vi "PvgeneratorOP600.vi"(8 "errin":errorcluster, 10 "network":path, 11 "path in":path) -> (0 "sortie d'erreur":errorcluster caption="errout", 1 "network out":path, 2 "tout bon":bool, 3 "Chaîne":string)   [LabVIEW 2020]
uses:
  VG/IS30%.vi
  VG/PN.vi
  SubVI/OP600ZP_VGConf.vi
panel:
  out "Tab1":string[][](array[string])
  out "nombre de remplacements":i32
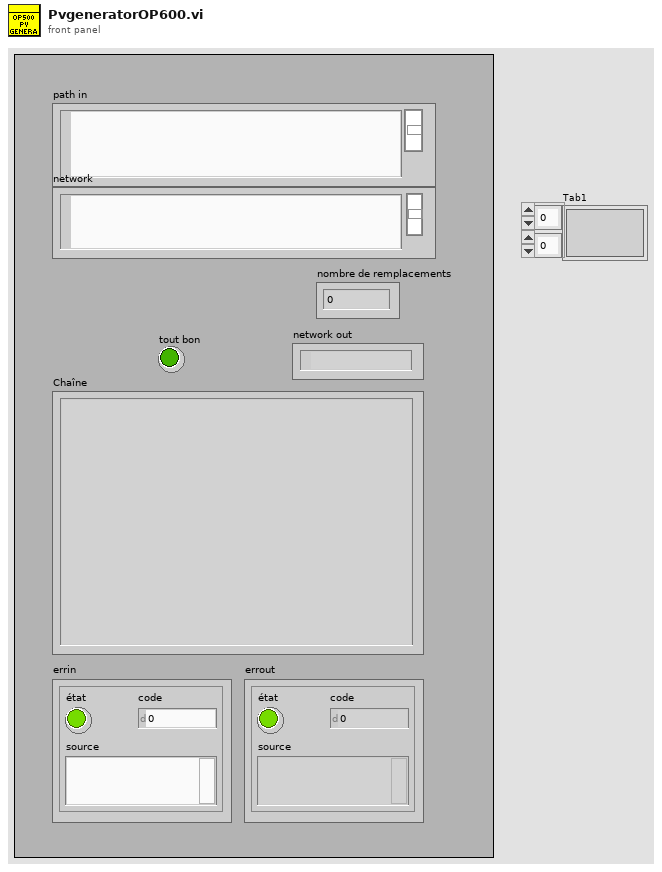
[diagram p1: front panel]
types:
  T1 = enum16{"open", "replace", "create", "open or create", "replace or create", "replace or create with confirmation"}
  T2 = cluster{string, string, string, string, string, string, string, string, string, string}
  T3 = cluster{string, string, string, string, string, string, string, string}
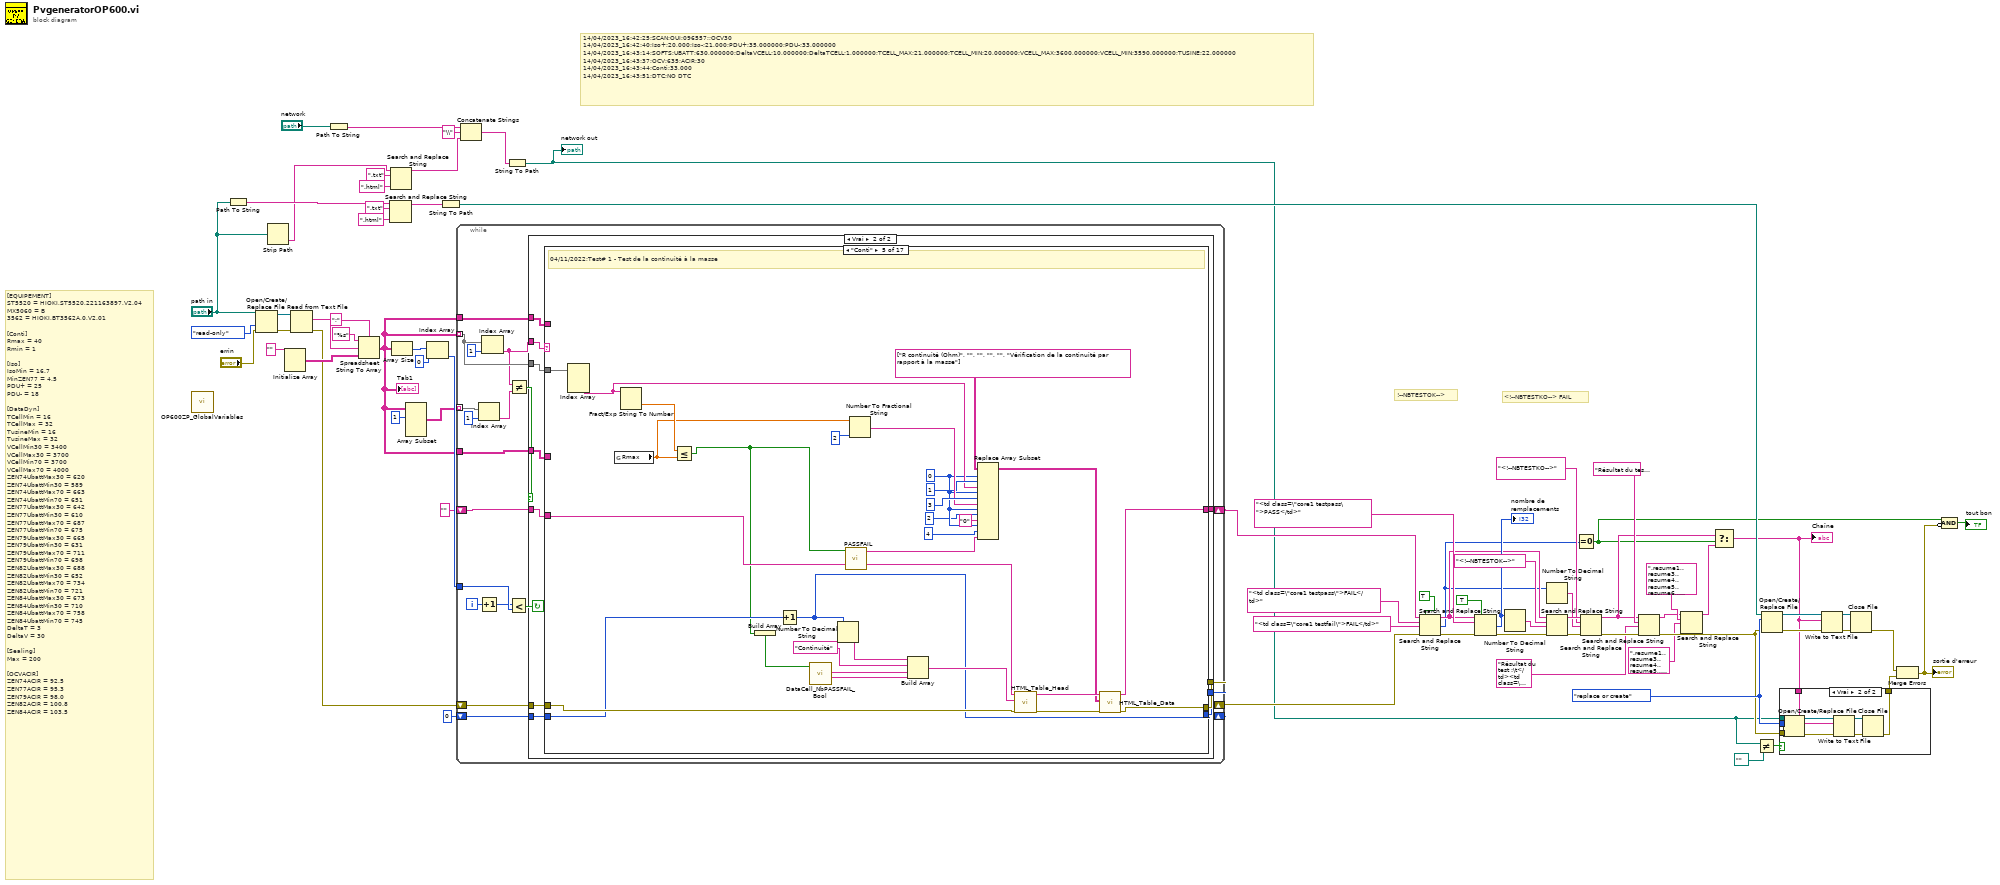
[diagram p0: block diagram]
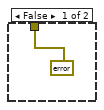
[diagram p2: hidden frame]
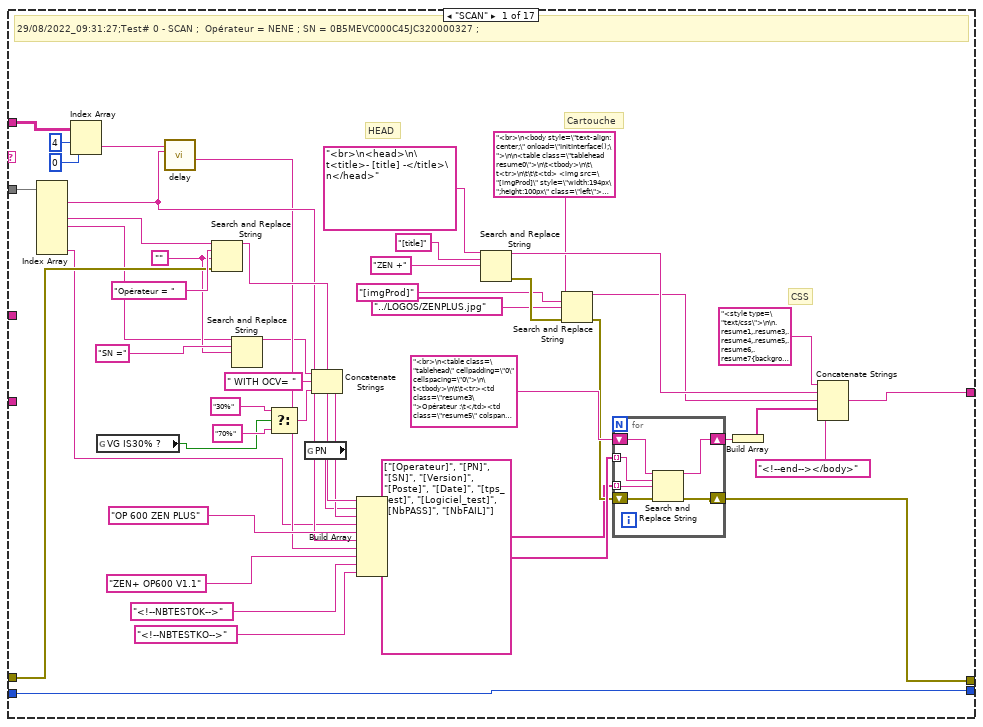
[diagram p4: hidden frame]
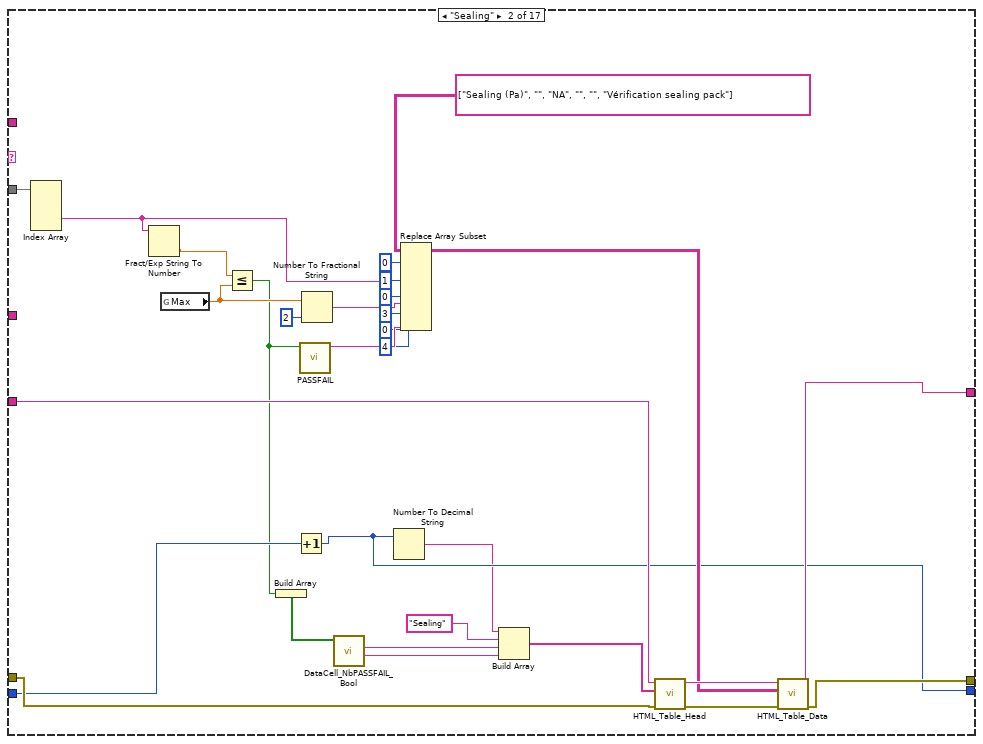
[diagram p5: hidden frame]
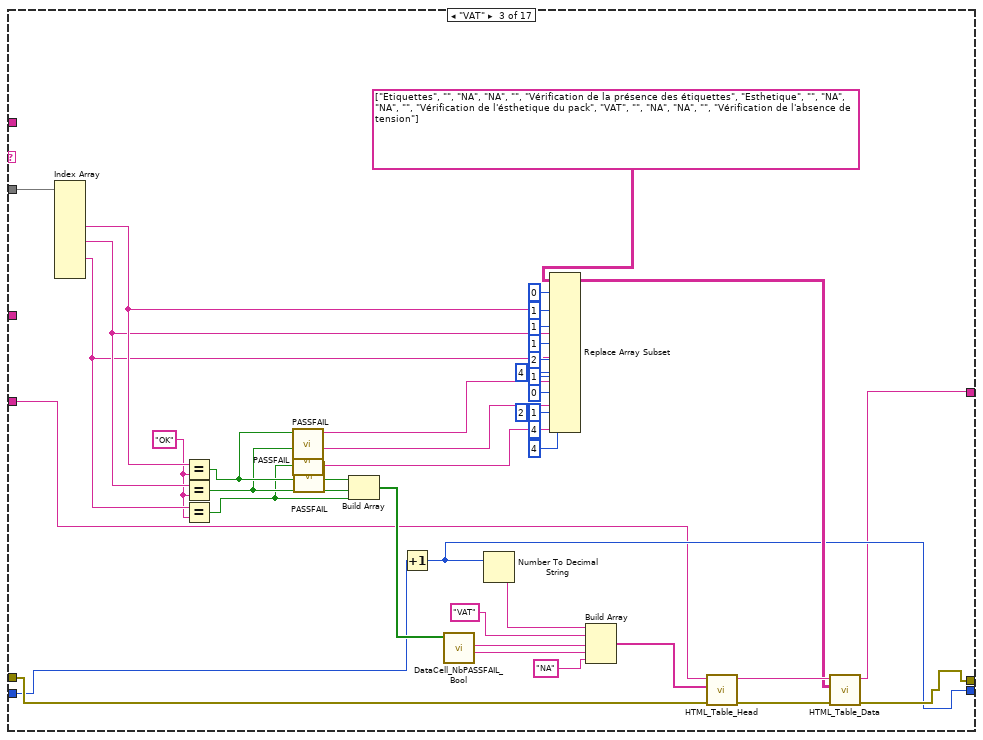
[diagram p6: hidden frame]
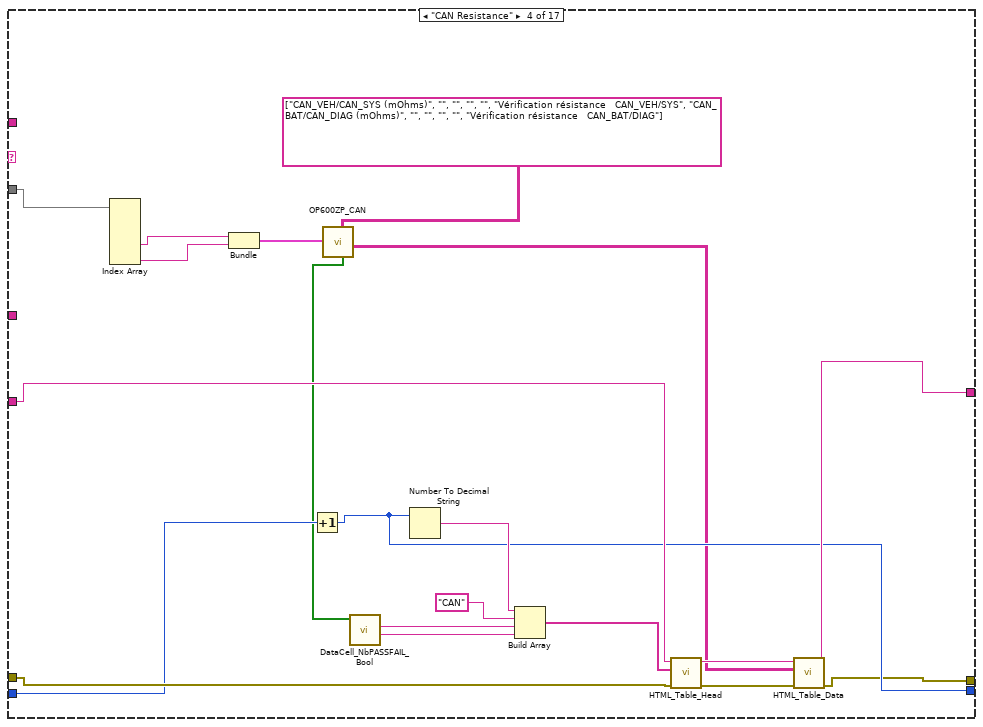
[diagram p7: hidden frame]
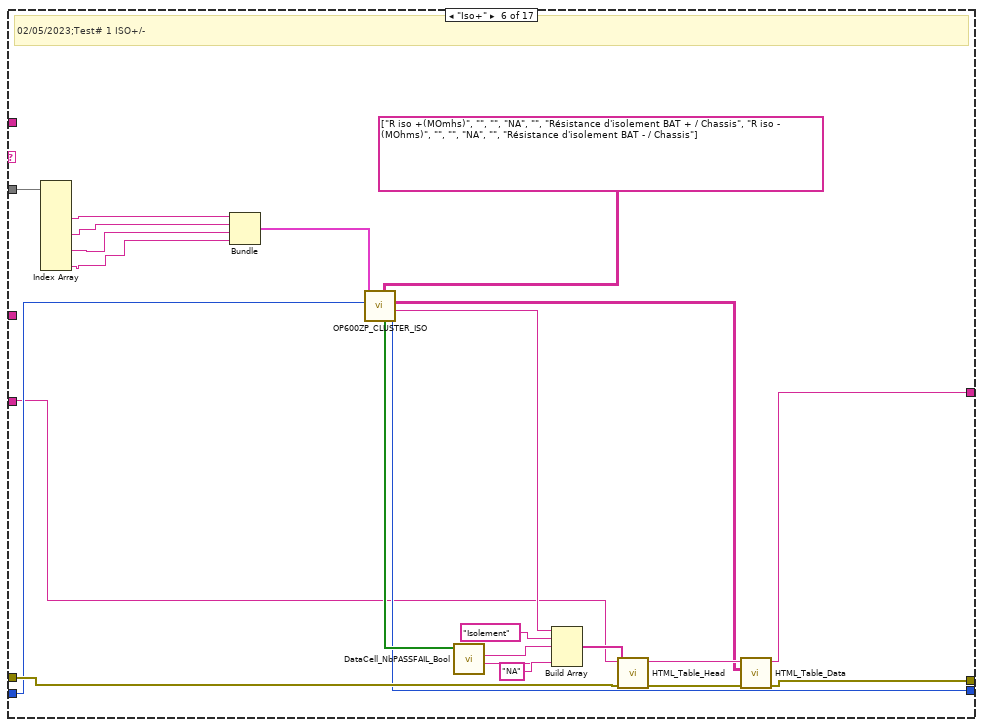
[diagram p8: hidden frame]
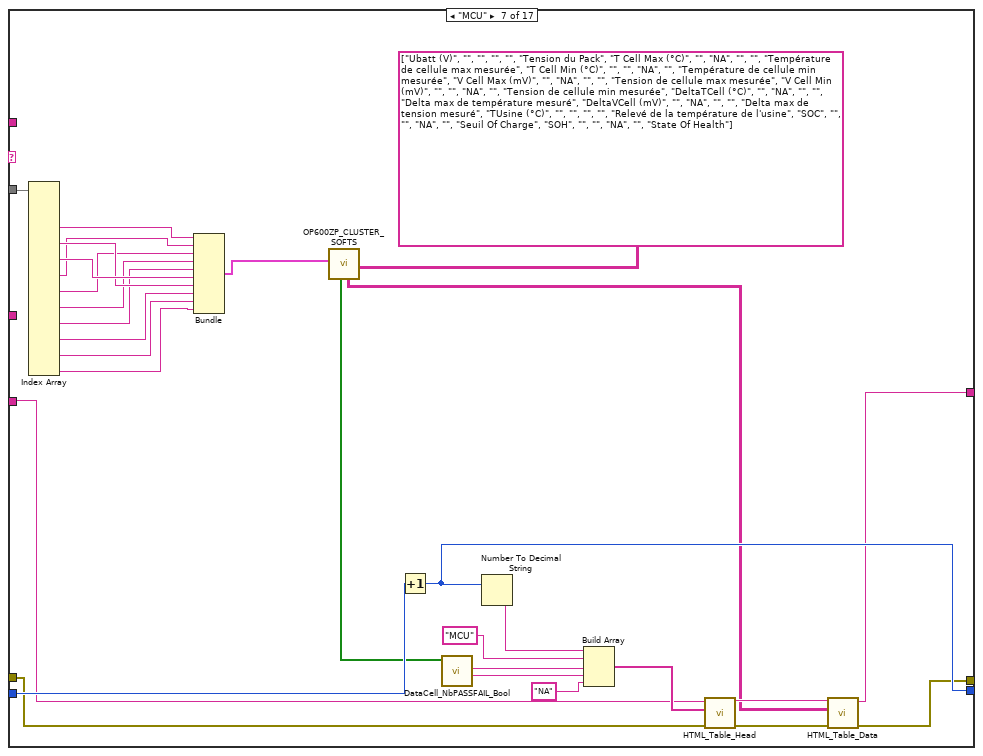
[diagram p9: hidden frame]
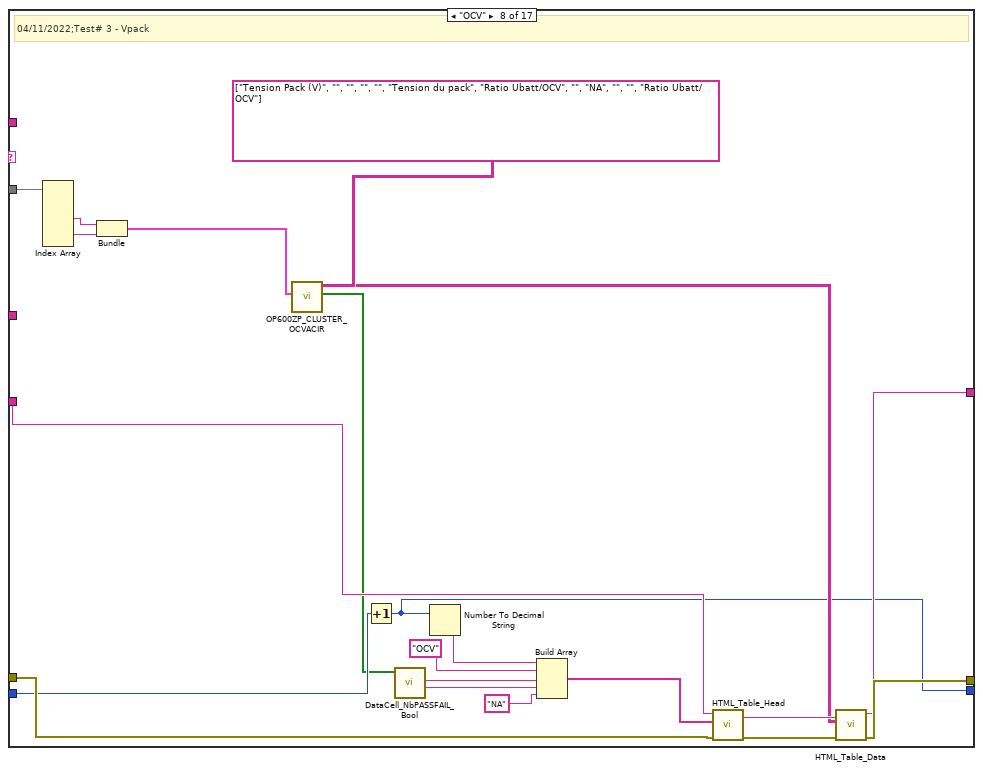
[diagram p10: hidden frame]
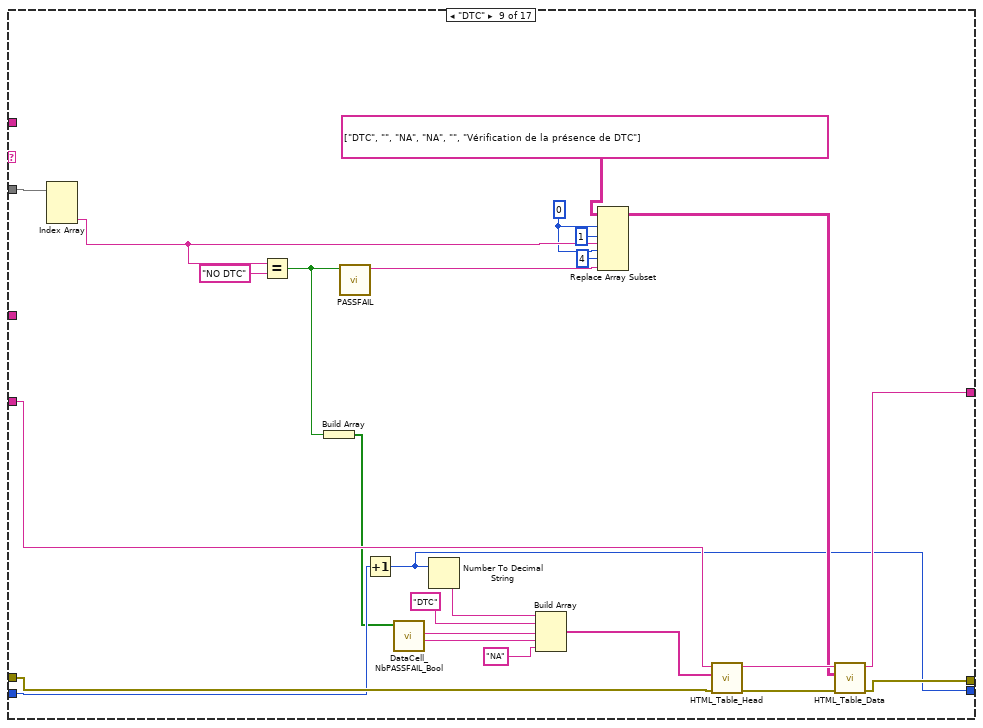
[diagram p11: hidden frame]
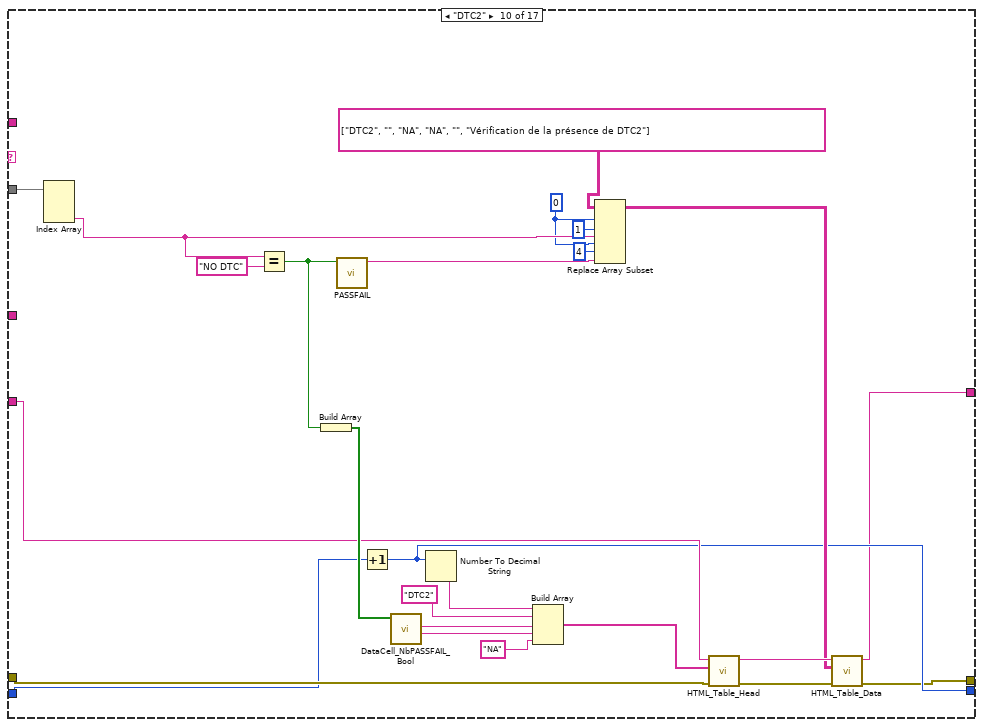
[diagram p12: hidden frame]
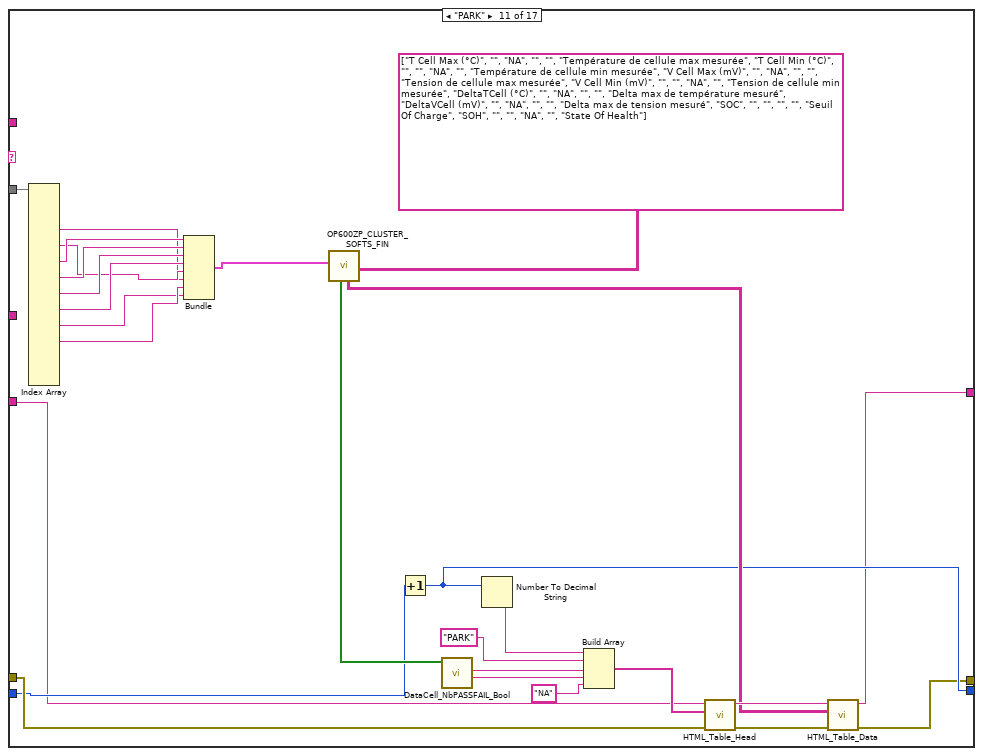
[diagram p13: hidden frame]
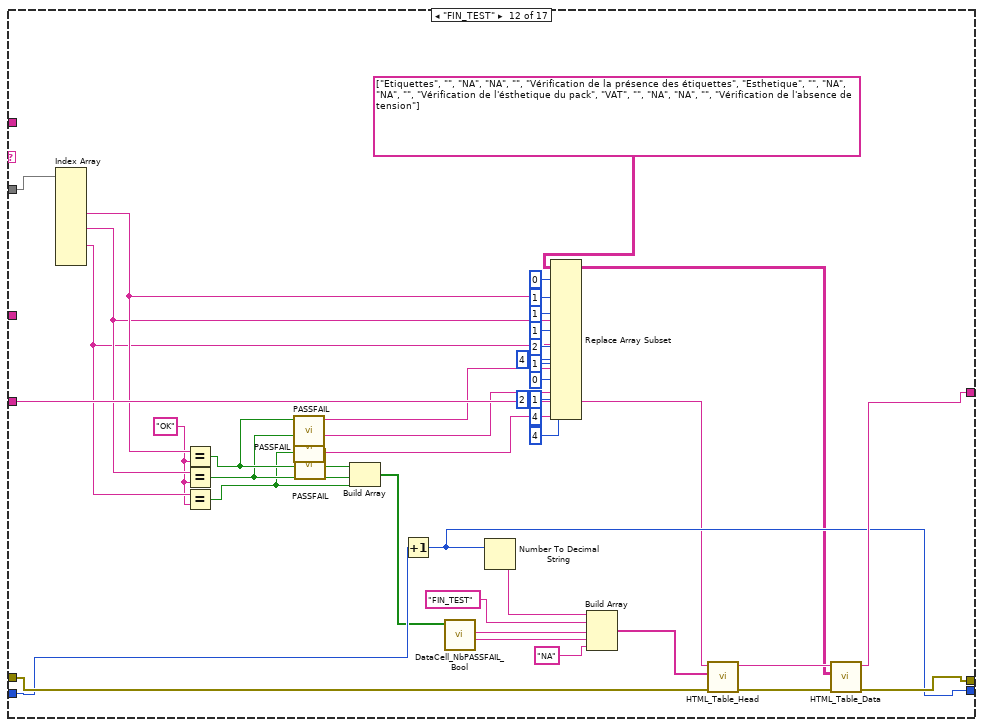
[diagram p14: hidden frame]
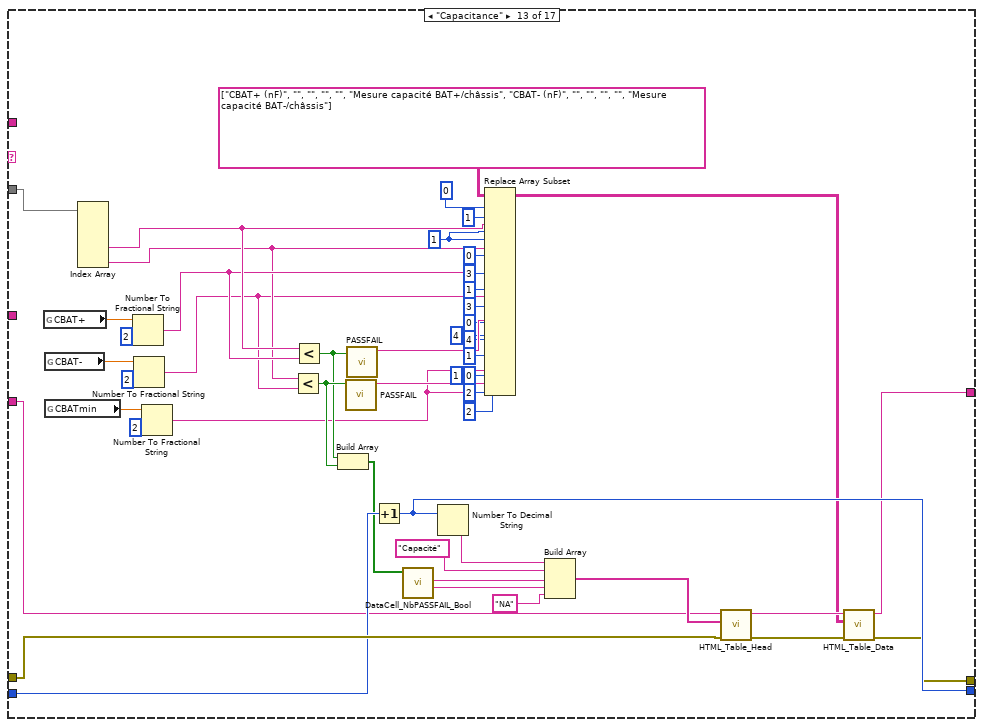
[diagram p15: hidden frame]
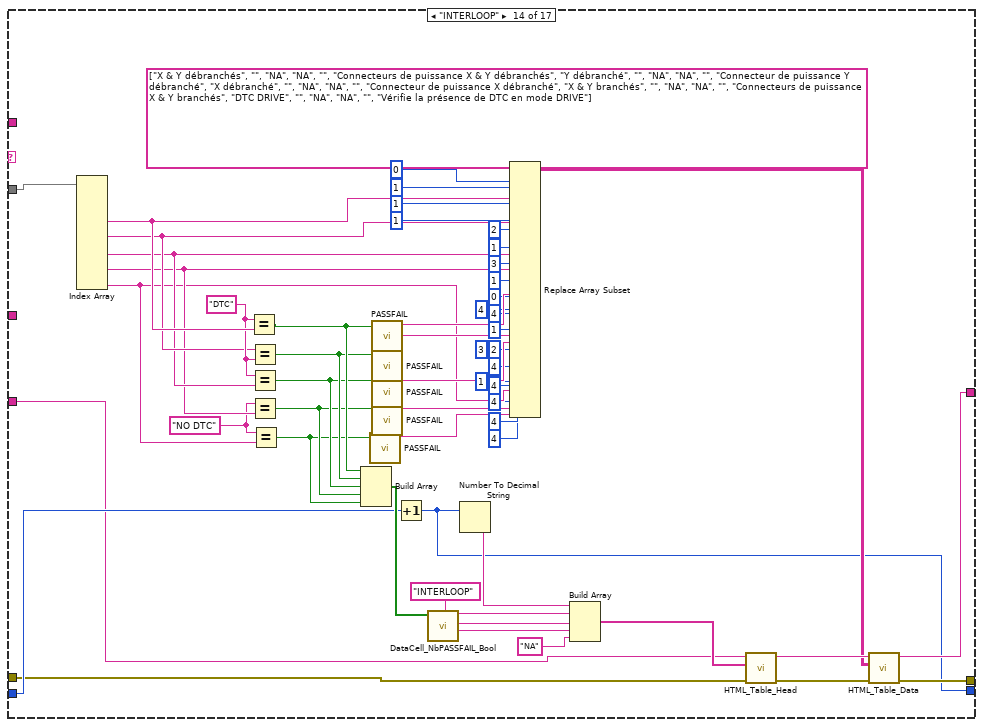
[diagram p16: hidden frame]
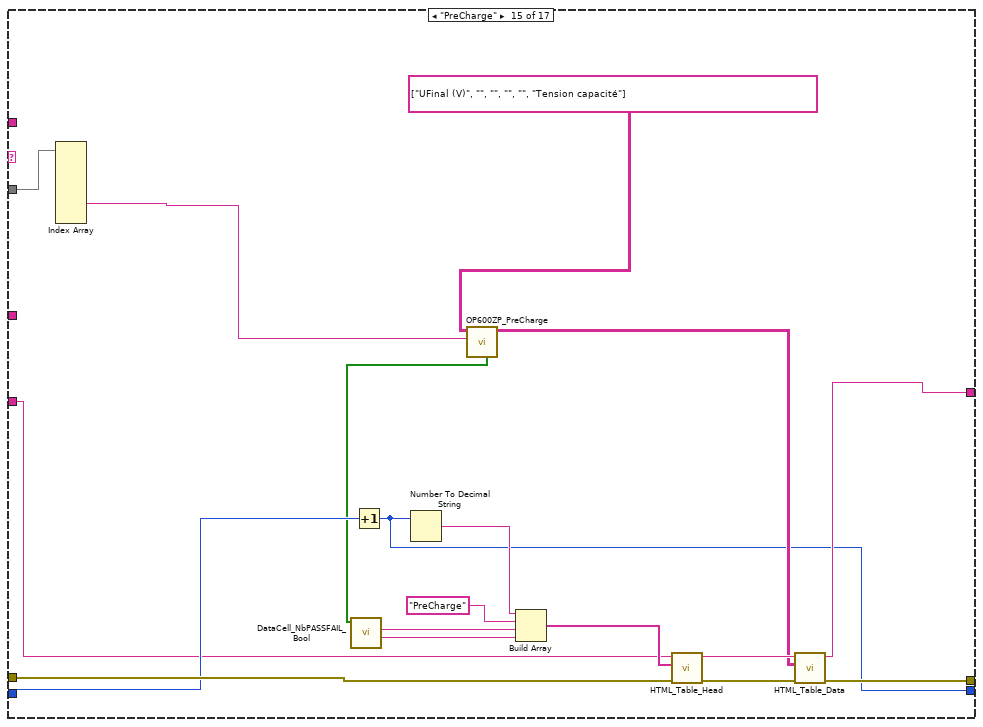
[diagram p17: hidden frame]
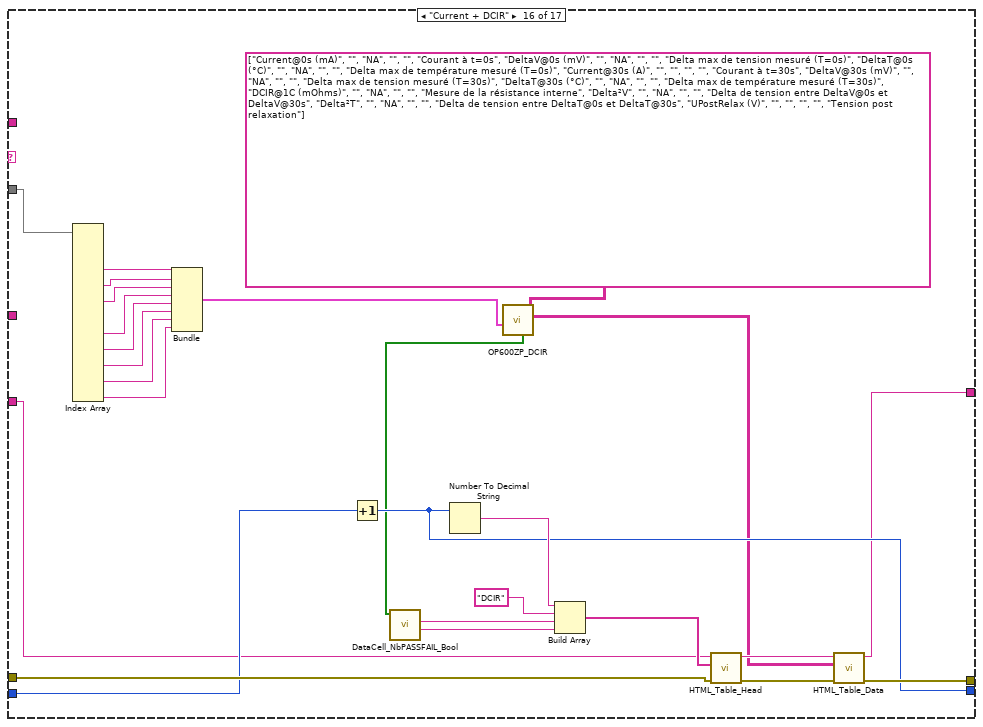
[diagram p18: hidden frame]
diagram:
  w32 = T1."replace or create" ("opération (0 : open)")
  # "14/04/2023_16:42:25;SCAN;OUI;096557;;OCV30\n14/04/2023_16:42:40;Iso+;20,000;Iso-;21,000;PDU+;35,000000;PDU-;33,000000\n14/04/2023_16:43:14;SOFTS;UBATT;630,000000;DeltaVCELL;10,000000;DeltaTCELL;1,000000;TCELL_MAX;21,000000;TCELL_MIN;20,000000;VCELL_MAX;3600,000000;VCELL_MIN;3590,000000;TUSINE;22,000000\n14/04/2023_16:43:37;OCV;635;ACIR;30\n14/04/2023_16:43:44;Conti;33,000\n14/04/2023_16:43:51;DTC;NO DTC"
  # "[EQUIPEMENT]\nST5520 = HIOKI,ST5520,221163897,V2.04\t\nMX5060 = B\n3562 = HIOKI,BT3562A,0,V2.01\n\n[Conti]\nRmax = 40\nRmin = 1\n\n[Iso]\nIsoMin = 16.7\nMinZEN77 = 4.5\nPDU+ = 25\nPDU- = 18\n\n[DataDyn]\nTCellMin = 16\nTCellMax = 32\nTusineMin = 16\nTusineMax = 32\nVCellMin30 = 3400\nVCellMax30 = 3700\nVCellMin70 = 3700\nVCellMax70 = 4000\nZEN74UbattMax30 = 620\nZEN74UbattMin30 = 589\nZEN74UbattMax70 = 663\nZEN74UbattMin70 = 651\nZEN77UbattMax30 = 642\nZEN77UbattMin30 = 610\nZEN77UbattMax70 = 687\nZEN77UbattMin70 = 675\nZEN79UbattMax30 = 665\nZEN79UbattMin30 = 631\nZEN79UbattMax70 = 711\nZEN79UbattMin70 = 698\nZEN82UbattMax30 = 688\nZEN82UbattMin30 = 652\nZEN82UbattMax70 = 734\nZEN82UbattMin70 = 721\nZEN84UbattMax30 = 673\nZEN84UbattMin30 = 710\nZEN84UbattMax70 = 758\nZEN84UbattMin70 = 745\nDeltaT = 3\nDeltaV = 30\n\n[Sealing]\nMax = 200\n\n[OCVACIR]\nZEN74ACIR = 92.5\nZEN77ACIR = 95.3\nZEN79ACIR = 98.0\nZEN82ACIR = 100.8\nZEN84ACIR = 103.5"
  # "<!--NBTESTKO--> FAIL"
  # "!--NBTESTOK-->"
  n1 = call "OP600ZP_GlobalVariables.vi"() -> ()  [unwired: 12 in]
  n2 = Path To String(path="path in") -> (string=w54:string)
  n3 = Open/Create/Replace File(file path (use dialog)="path in", error in="errin", access (0:read/write)=enum16{"read/write", "read-only", "write-only"}."read-only" ("accès (0 : read/write)")) -> (refnum out=w55:refnum<file>, error out=w72:errorcluster)  [unwired: 3 in, 1 out]
  n4 = Strip Path(path="path in") -> (name=w13:string)  [unwired: 1 out]
  n5 = Initialize Array("") -> (w70:string[][])  [unwired: 2 in]
  n6 = Read from Text File(file (use dialog)=w55, error in=w72) -> (text=w68:string, error out=w60:errorcluster)  [unwired: 2 in, 2 out]
  n7 = Path To String(path="network") -> (string=w12:string)
  n8 = Spreadsheet String To Array(delimiter (Tab)=";" ("séparateur (Tabulation)"), format string="%s" ("chaîne de format"), spreadsheet string=w68, array type (2D Dbl)=w70) -> (array=w3:string[][])
  "Tab1" <- w3
  n9 = Search and Replace String(input string=w54, search string=".txt" ("chaîne recherchée"), replace string=".html" ("chaîne de remplacement (\"\")")) -> (result string=w51:string)  [unwired: 5 in, 3 out]
  n10 = Search and Replace String(input string=w13, search string=".txt" ("chaîne recherchée"), replace string=".html" ("chaîne de remplacement (\"\")")) -> (result string=w10:string)  [unwired: 5 in, 3 out]
  n11 = Array Size(array=w3) -> (size(s)=w66:i32[])
  n12 = Array Subset(array=w3, index (row)=1 ("indice")) -> (w1:string[][])  [unwired: 3 in]
  n13 = Index Array(array=w66, index=0 ("indice")) -> (element=w64:i32)
  n14 = String To Path(string=w51) -> (path=w50:path)
  n15 = while {
    tunnel: w64 -> [w91]
    tunnel: w3 -> [w88] mode=indexing
    shift-right: [w87] -> w47
    shift-left: w60 -> [w86]
    shift-right: [w80] -> w49
    shift-left: "" -> [w85]
    shift-right: [w83] -> _
    shift-left: 0 -> [w84]
    tunnel: w3 -> [w82]
    tunnel: w3 -> [w79]
    tunnel: w1 -> [w77] mode=indexing
    i -> [w92]
    stop <- w90 continue-if-true
    n16 = Index Array(array=w77, index=1 ("indice")) -> (element=w76:string)
    n17 = Increment(x=w92) -> (x+1=w81:i32)
    n18 = Index Array(array=w88, index=1 ("indice")) -> (element=w75:string)
    n19 = Less?(x=w81, y=w91) -> (x < y?=w90:bool)
    n20 = Not Equal?(x=w75, y=w76) -> (x != y?=w74:bool)
    n21 = case shown="Vrai" w74 {
      tunnel: w88 -> [_ w105]
      tunnel: [w94 w97] -> w87
      tunnel: w86 -> [w94 w104]
      tunnel: w85 -> [w95 w103]
      tunnel: w84 -> [w93 w102]
      tunnel: [w93 w96] -> w83
      tunnel: w82 -> [_ w101]
      tunnel: [w95 w98] -> w80
      tunnel: w75 -> [_ w100]
      tunnel: w79 -> [_ w99]
      frame False {
      }
      frame True {
        n22 = case shown="\"Conti\"" w100 {
          tunnel: w104 -> [w150 w182 w192 w241 w271 w294 w318 w343 w368 w383 w416 w458 w504 w527 w580 w607 w618]
          tunnel: w105 -> [w152 w188 w189 w235 w272 w295 w330 w344 w361 w381 w417 w468 w516 w571 w589 w615 _]
          tunnel: [w129 w181 w195 w236 w270 w293 w316 w342 w367 w378 w412 w457 w499 w529 w575 w606 w618] -> w97
          tunnel: w103 -> [_ w175 w193 w238 w269 w285 w315 w341 w362 w380 w414 w453 w501 w526 w578 w593 w616]
          tunnel: w102 -> [w128 w177 w191 w240 w268 w292 w322 w340 w366 w382 w415 w454 w503 w528 w579 w605 w617]
          tunnel: [w128 w174 w194 w237 w267 w286 w321 w331 w352 w379 w413 w455 w502 w525 w574 w604 w617] -> w96
          tunnel: w101 -> [_ _ _ _ _ _ _ _ _ _ _ _ _ _ _ _ _]
          tunnel: w99 -> [w121 _ _ _ _ _ _ _ _ _ _ _ _ _ _ _ _]
          tunnel: [w127 w176 w190 w239 w266 w291 w320 w339 w363 w377 w411 w456 w498 w530 w576 w602 w616] -> w98
          frame "SCAN" {
            w123 = ""
            # "Cartouche"
            # "HEAD"
            # "CSS"
            # "29/08/2022_09:31:27;Test# 0 - SCAN ;  Opérateur = NENE ; SN = 0B5MEVC000C45JC320000327 ;"
            n23 = Index Array(array=w152) -> (element #1=w117:string, element #3=w126:string, element #4=w122:string, element #7=w106:string)  [unwired: 7 in, 3 out]
            n24 = Index Array(array=w121, index (row)=4, index (col)=0 ("disabled index (col)")) -> (element=w118:string)
            n25 = global read "IS30%.vi" "VG IS30% ?"() -> (w108:bool)
            n26 = call "delay.vi"("String"=w117, "String 2"=w118) -> ("Delay calculé"=w116:string)  [unwired: 9 in]
            n27 = Search and Replace String(input string=w126, search string="Opérateur = " ("chaîne recherchée"), replace string=w123, error in=w150) -> (result string=w125:string)  [unwired: 4 in, 3 out]
            n28 = Search and Replace String(input string=w122, search string="SN =" ("chaîne recherchée"), replace string=w123) -> (result string=w114:string)  [unwired: 5 in, 3 out]
            n29 = Select(t="30%" ("y"), s=w108, f="70%" ("y")) -> (s? t:f=w111:string)
            n30 = global read "PN.vi" "PN"() -> (w107:string)
            n31 = Concatenate Strings(w114, " WITH OCV= " ("chaîne"), w111) -> (w113:string)
            n32 = Build Array(w125, w107, w113, w106, "OP 600 ZEN PLUS" ("chaîne"), w117, w116, "ZEN+ OP600 V1.1" ("chaîne"), "<!--NBTESTOK-->" ("chaîne"), "<!--NBTESTKO-->" ("chaîne")) -> (w130:string[])
            n33 = Search and Replace String(input string="<br>\n<head>\n\t<title>- [title] -</title>\n</head>", search string="[title]" ("chaîne recherchée"), replace string="ZEN +" ("Title")) -> (result string=w146:string, error out=w145:errorcluster)  [unwired: 5 in, 2 out]
            n34 = Search and Replace String(input string="<br>\n<body style=\"text-align: center;\" onload=\"InitInterface();\">\n\n<table class=\"tablehead resume0\">\n\t<tbody>\n\t\t<tr>\n\t\t\t<td> <img src=\"[imgProd]\" style=\"width:194px\";height:100px\" class=\"left\"></td>\n\t\t\t<td> <div class=\"center\">PROCES VERBAL DE TEST AUTOMATIQUE</div><div class=\"center\">Zen Plus OP 600</div><br class=\"center\"><div class=\"center\">Forseepower</div></td>\n\t\t\t<td> <img src=\"../LOGOS/LOGO FORSEE.png\" style=\"width:194px\"  class=\"right\"></td>\n\t\t</tr>\n\t</tbody>\n</table>", search string="[imgProd]", replace string="../LOGOS/ZENPLUS.jpg" ("imgProd"), error in=w145) -> (result string=w143:string, error out=w140:errorcluster)  [unwired: 4 in, 2 out]
            n35 = for {
              shift-right: [w157] -> w139
              shift-left: "<br>\n<table class=\"tablehead\" cellpadding=\"0\" cellspacing=\"0\">\n\t<tbody>\n\t\t<tr><td class=\"resume3\">Opérateur :\t</td><td class=\"resume5\" colspan=\"3\">[Operateur]</td></tr>\n\t\t<tr><td class=\"resume3\">PN : </td><td class=\"resume5\" colspan=\"3\">[PN]</td></tr>\n\t\t<tr><td class=\"resume3\">SN : </td><td class=\"resume5\" colspan=\"3\">[SN]</td></tr>\n\t\t<tr><td class=\"resume3\">Version : </td><td class=\"resume5\" colspan=\"3\">[Version]</td></tr>\n\t\t<tr><td class=\"resume3\">Poste : </td><td class=\"resume5\" colspan=\"3\">[Poste]</td></tr>\t\t\n\t\t<tr><td class=\"resume3\">Date du test : </td><td class=\"resume5\" colspan=\"3\">[Date]</td></tr>\n\t\t<tr><td class=\"resume3\">Temps de test : </td><td class=\"resume5\" colspan=\"3\">[tps_test]</td></tr>\n\t\t<tr><td class=\"resume3\">Logiciel de test :\t</td><td class=\"resume5\" colspan=\"3\">[Logiciel_test]</td></tr>\n\t\t<tr><td class=\"resume3\">Résultat du test :\t</td><td class=\"resume5\" colspan=\"3\"><div><span style=\"float:left\" id=\"result\"><font size = \"5pt\" color=\"green\"><b>CONFORME</b></font><b><font size = \"5pt\"> ( </font><font size = \"5pt\" color=\"green\">[NbPASS] PASS </font>  <font size = \"5pt\"> / </font><font size = \"5pt\" color=\"red\">[NbFAIL] FAIL</font> <font size = \"5pt\"> ) </font></b></span></div></td></tr>\n\t</tbody>\n</table>" -> [w158]
              tunnel: string[] ["[Operateur]", "[PN]", "[SN]", "[Version]", "[Poste]", "[Date]", "[tps_test]", "[Logiciel_test]", "[NbPASS]", "[NbFAIL]"] -> [w154] mode=indexing
              tunnel: w130 -> [w153] mode=indexing
              shift-right: [w155] -> w129
              shift-left: w140 -> [w156]
              n36 = Search and Replace String(input string=w158, search string=w154, replace string=w153, error in=w156) -> (result string=w157:string, error out=w155:errorcluster)  [unwired: 4 in, 2 out]
            }
            n37 = Build Array(w139) -> (w138:string[])
            n38 = Concatenate Strings("<style type=\"text/css\">\n\n.resume1,.resume3,.resume4,.resume5,.resume6,.resume7{background-color:#e6feef;padding:7px;border:1px solid black;}\n.resume0{border:1px solid black;background-color:#e6feef;font-weight: bold;padding:0px;text-align: center;}\n.resume1{width:350px;text-align:right;font-weight:bold;}\n.resume3{width:350px;text-align:right;border-top:0px solid black;font-weight:bold;}\n.resume4{border-left:0px solid black;width:290px;}\n.resume5{width:290px;border-left:0px solid black;border-top:0px solid black;}\n.resume6{border-left:0px solid black;width:60px;}\n.resume7{border-left:0px solid black;border-top:0px solid black;width:60px;}\n.title1{text-align: left;background-color:#e6f4fe;padding:10px;border:1px solid #101010;}\n.title2{width: 30px;text-align: center;background-color:#e6f4fe;padding:1px;border:1px solid #101010;border-left:0px solid black;font-weight: bold;}\n.title2 a:link{text-decoration:none;}\n.entete0,.entete1,.entete2,.time2{text-align: center;background-color:#feeec9;padding:7px;border:1px solid black;font-weight: bold;}\n.entete0{width:45px;border-right:0px solid black;}\n.entete1{width:505px;}\n.entete2{width:95px;border-right:0px solid black;}\n.time2{border-left:0px solid black;width:145px;font-size:11px;}\n.core0,.core1,.core2,.core3,.core4,.time{text-align: center;background-color:#fafed3;padding:7px;border:1px solid black;}\n.core0, .core1,.core3,.core4{width:95px;border-top:0px solid black;border-right:0px solid black;}\n.core0{width:45px;}\n.core2{border-top:0px solid black;width:505px;}\n.core3{width:200px;}\n.core4{width:300px;}\n.time{width:145px;border-top:0px solid black;border-left:0px solid black;font-size:11px;}\n.false .core0,.false .core1,.false .core2,.false .core3,.false .core4,.false .time{background-color:#f4f4f4;}\n.false .entete0,.false .entete1,.false .entete2,.false .time2{background-color:#dadada;}\n.false .title1,.false .title2,.false .resultentete .testpass,.false .resultentete .testfail,.false .resultentete .testtime{background-color:#c5cac9;color: blue;}\n.false .title2 a:link{text-decoration:none;color: blue;}\n.comment1,.comment2,.time3{width: 890px;background-color:#e9e8e9;padding:7px;border:1px solid black;border-top:0px solid black;text-align:left;}\n.comment2{border-right:0px solid black;width: 45px;text-align: center;}\n.time3{width: 145px;border-left:0px solid black;font-size:11px;}\n.fixe1{background: -moz-linear-gradient(center top , #101010 10%, #555555 80%) repeat scroll 0 0 transparent;background: -webkit-gradient(linear, left top, left bottom, from(#101010), to(#555555));border:2px solid orange;position : fixed;margin-top:20px;display:none;overflow-y:scroll;max-height:350px;text-shadow: 0px 0px 0 #333333;text-align:left;font-size:10px;padding:10px;margin-left:-162px;border-radius: 15px 15px 15px 15px;}\n.menufixe, .menufixelock{background: -moz-linear-gradient(center top , #101010 80%, transparent 20%) repeat scroll 0 0 transparent;background: -webkit-gradient(linear, left top, left bottom, from(#101010), color-stop(0.65, #101010), to(transparent)) repeat scroll 0 0 transparent;margin: -52px 0px 0px -9px;width:100%;position:fixed;height:55px;-moz-transition: margin 1s;-webkit-transition: margin 1s;}\n.menufixelock, .menufixe:hover{margin: -9px 0px 0px -9px;}\n.lockmenu, .separation,.separationmenu{text-align:center;background: -moz-linear-gradient(center top , #555555 10%, #111111 80%) repeat scroll 0 0 transparent;background: -webkit-gradient(linear, left top, left bottom, from(#555555), to(#111111));border: 1px solid white;border-radius: 10px 10px 10px 10px;box-shadow: 0 -1px 1px #555555 inset;color: #999999;font-weight: bold;width: 100px;padding: 2px;text-decoration: none;}\n.tablehead{width: 1000px;font-family: Verdana;font-size: 12px;margin-left: auto;margin-right: auto;}\n.tablenull{font-family: Verdana;font-size: 11px;margin-left: auto;margin-right: auto;}\n.separationmenu:hover div{display: inline;}\n.lockmenu:hover, .separation:hover,.separationmenu:hover{border: 1px solid orange;cursor:pointer;}\n.lockmenu:hover{border: 1px solid red;cursor:pointer;}\n.separationright{padding:10px;}\ndiv a:link{text-decoration:none;color:#cbcbcb;}\ndiv a:hover{text-decoration:underline;color:#cbcbcb;}\nspan a:link{text-decoration:none;color:#cbcbcb;}\nspan a:hover{text-decoration:none;color:#cbcbcb;}\n.false{color: blue;}\n.testpass{color: green;font-weight: bold;}\n.testfail{color: red;font-weight: bold;}\n.testtime{color: blue;font-weight: bold;}\n.resultentete{font-weight: bold;font-size: 11px;min-width: 200px;text-align:right;}\n.infohard{border: 1px solid black;background-color: white;text-align: center;width: 16px;height: 16px;border-radius: 5px;font-weight: bold;box-shadow: 0 -1px 2px #555555 inset;}\n.infohard:hover{background-color:#feeec9;cursor:pointer;}\n.footerhard{padding-top:30px;}\n.confighard{font-size:10px;width:110px;}\n.circlemain{margin-left:auto;margin-right:auto;}\n.circletext,.circleform{padding-top: 3px;text-align:center;font-size: 10px;width:200px;}\n.circleform{padding-bottom: 3px;padding-top: 1px;}\n.circle{border: 1px solid black;border-collapse: collapse;border-radius: 15px;box-shadow: 1px 1px 0 #505050;height: 15px;width: 15px;display:inline-block;}\n.bookmarkon, .bookmarkoff{background-color: yellow;border: 1px solid black;border-collapse: collapse;border-radius: 10px 10px 10px 10px;box-shadow: 1px 1px 0 #505050;height: 12px;width: 12px;position: absolute;margin-left:22px;cursor: help;}\n.bookmarkoff{background-color: transparent;border: 1px solid #CECECE;box-shadow: none;cursor: copy;}\n.false .bookmarkoff{background-color: transparent;border: 1px solid #E6E1E1;box-shadow: none;cursor: copy;}\n.bookmarkmaster{height: 15px;margin-right: 12px;width: 60px;}\n.bookmarkmaster:hover .bookmarkprev,.bookmarkmaster:hover .bookmarksuiv{display:block;}\n.bookmarkprev, .bookmarksuiv {cursor: pointer;font-size: 25px;font-weight: bold;margin-top: -10px;position: absolute;display:none;}\n.bookmarkprev{margin-left: 2px;}\n.bookmarksuiv{margin-left: 43px;}\n.plus, .moins{background-color: #F4F4F4;border: 1px solid #848484;border-radius: 20px;color: #848484;font-family: arial;font-size: 16px;font-weight: bold;height: 20px;margin-left: 4px;text-align: center;width: 20px;}\n.moins{font-size: 15px;}\n.plus:hover, .moins:hover{background-color: #DADADA;border: 1px solid black;color: black;cursor:pointer;}\n.backtothetop {position: fixed; right: 50%; margin-right: -555px; bottom: 10px; font-size: 35px; font-weight: bold; border: 1px solid #7D7B91; width: 40px; height: 40px; line-height:52px; text-align: center;border-radius: 8px; opacity: 0.25; background-color: #F5F5F5; color:#7D7B91;}\n.backtothetop:hover {opacity: 1; cursor:pointer;}\n.libversion {font-size: 8px;font-weight: normal;padding-right: 10px;text-align: right;}\n.lockmenu {width: 18px;font-size: 12px;}\n.left {display: block; margin-left: 1px;margin-right: auto;}\n.right {display: block; margin-right: 1px;margin-left: auto;}\n.center {display: block; margin-left: auto;margin-right: auto;}\n\n</style>", w146, w143, w138, "<!--end--></body>") -> (w127:string)
          }
          frame "Sealing" {
            n39 = Index Array(array=w188) -> (element #3=w171:string)  [unwired: 4 in, 3 out]
            n40 = Fract/Exp String To Number(string=w171) -> (number=w170:dbl)  [unwired: 3 in, 1 out]
            n41 = global read "OP600ZP_VGConf.vi" "Max"() -> (w167:dbl)
            n42 = Less Or Equal?(x=w170, y=w167) -> (x <= y?=w162:bool)
            n43 = Build Array(w162) -> (w183:bool[])
            n44 = Increment(x=w177) -> (x+1=w174:i32)
            n45 = call <vilib>:"PASSFAIL.vi"("E"=w162) -> ("S"=w161:string)  [unwired: 10 in]
            n46 = Number To Fractional String(number=w167, precision (6)=i16 2 ("précision (6)")) -> (F-format string=w165:string)  [unwired: 2 in]
            n47 = call <vilib>:"DataCell_NbPASSFAIL_Bool.vi"("Tableau en entrée"=w183) -> ("Chaîne"=w168:string, "Chaîne 2"=w169:string)  [unwired: 8 in, 1 out]
            n48 = Number To Decimal String(number=w174) -> (decimal integer string=w173:string)  [unwired: 1 in]
            n49 = Replace Array Subset(array=string[][] [["Sealing (Pa)", "", "NA", "", "", "Vérification sealing pack"]] ("Tableau"), new element #1=w171, index (row) #1=0 ("indice (ligne)"), index (col) #1=1 ("indice désactivé (col)"), new element #2=w165, index (row) #2=0 ("indice (ligne)"), index (col) #2=3 ("indice désactivé (col)"), new element #3=w161, index (row) #3=0 ("indice (ligne)"), index (col) #3=4 ("indice désactivé (col)")) -> (w180:string[][])
            n50 = Build Array(w173, "Sealing" ("élément"), w169, w168) -> (w186:string[])
            n51 = call "HTML_Table_Head.vi"("entrée d'erreur (pas d'erreur)"=w182, "Tableau"=w186, "chaîne en entrée"=w175) -> ("sortie d'erreur"=w185:errorcluster, "result string"=w184:string)  [unwired: 7 in]
            n52 = call "HTML_Table_Data.vi"("entrée d'erreur (pas d'erreur)"=w185, "Tableau"=w180, "chaîne en entrée"=w184) -> ("sortie d'erreur"=w181:errorcluster, "result string"=w176:string)  [unwired: 7 in]
          }
          frame "VAT" {
            w209 = "OK"
            n53 = Index Array(array=w189) -> (element #4=w212:string, element #6=w211:string, element #8=w210:string)  [unwired: 10 in, 7 out]
            n54 = Equal?(x=w212, y=w209) -> (x = y?=w207:bool)
            n55 = Equal?(x=w211, y=w209) -> (x = y?=w206:bool)
            n56 = Equal?(x=w210, y=w209) -> (x = y?=w205:bool)
            n57 = call <vilib>:"PASSFAIL.vi"("E"=w207) -> ("S"=w204:string)  [unwired: 10 in]
            n58 = call <vilib>:"PASSFAIL.vi"("E"=w206) -> ("S"=w203:string)  [unwired: 10 in]
            n59 = call <vilib>:"PASSFAIL.vi"("E"=w205) -> ("S"=w202:string)  [unwired: 10 in]
            n60 = Build Array(w207, w206, w205) -> (w208:bool[])
            n61 = Increment(x=w191) -> (x+1=w194:i32)
            n62 = call <vilib>:"DataCell_NbPASSFAIL_Bool.vi"("Tableau en entrée"=w208) -> ("Chaîne"=w221:string, "Chaîne 2"=w222:string)  [unwired: 8 in, 1 out]
            n63 = Number To Decimal String(number=w194) -> (decimal integer string=w225:string)  [unwired: 1 in]
            n64 = Replace Array Subset(array=string[][] [["Etiquettes", "", "NA", "NA", "", "Vérification de la présence des étiquettes"], ["Esthetique", "", "NA", "NA", "", "Vérification de l'ésthetique du pack"], ["VAT", "", "NA", "NA", "", "Vérification de l'absence de tension"]] ("Tableau"), new element #1=w212, index (row) #1=0 ("indice (ligne)"), index (col) #1=1 ("indice désactivé (col)"), new element #2=w211, index (row) #2=1 ("indice (ligne)"), index (col) #2=1 ("indice désactivé (col)"), new element #3=w210, index (row) #3=2 ("indice (ligne)"), index (col) #3=1 ("indice désactivé (col)"), new element #4=w204, index (row) #4=0 ("indice (ligne)"), index (col) #4=4 ("indice désactivé (col)"), new element #5=w203, index (row) #5=1 ("indice (ligne)"), index (col) #5=4 ("indice désactivé (col)"), new element #6=w202, index (row) #6=2 ("indice (ligne)"), index (col) #6=4 ("indice désactivé (col)")) -> (w219:string[][])
            n65 = Build Array(w225, "VAT" ("élément"), w222, w221, "NA" ("élément")) -> (w227:string[])
            n66 = call "HTML_Table_Head.vi"("entrée d'erreur (pas d'erreur)"=w192, "Tableau"=w227, "chaîne en entrée"=w193) -> ("sortie d'erreur"=w220:errorcluster, "result string"=w226:string)  [unwired: 7 in]
            n67 = call "HTML_Table_Data.vi"("entrée d'erreur (pas d'erreur)"=w220, "Tableau"=w219, "chaîne en entrée"=w226) -> ("sortie d'erreur"=w195:errorcluster, "result string"=w190:string)  [unwired: 7 in]
          }
          frame "CAN Resistance" {
            n68 = Index Array(array=w235) -> (element #4=w230:string, element #6=w229:string)  [unwired: 6 in, 4 out]
            n69 = Bundle(w230, w229) -> (w234:cluster{string, string})  [unwired: 1 in]
            n70 = Increment(x=w240) -> (x+1=w237:i32)
            n71 = call "OP600ZP_CAN.vi"("Tableau 3"=string[][] [["CAN_VEH/CAN_SYS (mOhms)", "", "", "", "", "Vérification résistance   CAN_VEH/SYS"], ["CAN_BAT/CAN_DIAG (mOhms)", "", "", "", "", "Vérification résistance   CAN_BAT/DIAG"]] ("Tableau"), "CAN_MESURES"=w234) -> ("Tableau 2"=w232:string[][], "Tableau"=w231:bool[])  [unwired: 8 in]
            n72 = call <vilib>:"DataCell_NbPASSFAIL_Bool.vi"("Tableau en entrée"=w231) -> ("Chaîne"=w242:string, "Chaîne 2"=w243:string)  [unwired: 8 in, 1 out]
            n73 = Number To Decimal String(number=w237) -> (decimal integer string=w245:string)  [unwired: 1 in]
            n74 = Build Array(w245, "CAN" ("élément"), w243, w242) -> (w248:string[])
            n75 = call "HTML_Table_Head.vi"("entrée d'erreur (pas d'erreur)"=w241, "Tableau"=w248, "chaîne en entrée"=w238) -> ("sortie d'erreur"=w247:errorcluster, "result string"=w246:string)  [unwired: 7 in]
            n76 = call "HTML_Table_Data.vi"("entrée d'erreur (pas d'erreur)"=w247, "Tableau"=w232, "chaîne en entrée"=w246) -> ("sortie d'erreur"=w236:errorcluster, "result string"=w239:string)  [unwired: 7 in]
          }
          frame "Conti" {
            w254 = 0 ("index (row)")
            # "04/11/2022;Test# 1 - Test de la continuité à la masse"
            n77 = Index Array(array=w272) -> (element #3=w257:string)  [unwired: 3 in, 2 out]
            n78 = global read "OP600ZP_VGConf.vi" "Rmax"() -> (w250:dbl)
            n79 = Fract/Exp String To Number(string=w257) -> (number=w252:dbl)  [unwired: 3 in, 1 out]
            n80 = Less Or Equal?(x=w252, y=w250) -> (x <= y?=w251:bool)
            n81 = Build Array(w251) -> (w264:bool[])
            n82 = Increment(x=w268) -> (x+1=w267:i32)
            n83 = call <vilib>:"DataCell_NbPASSFAIL_Bool.vi"("Tableau en entrée"=w264) -> ("Chaîne"=w262:string, "Chaîne 2"=w263:string)  [unwired: 8 in, 1 out]
            n84 = Number To Decimal String(number=w267) -> (decimal integer string=w274:string)  [unwired: 1 in]
            n85 = call <vilib>:"PASSFAIL.vi"("E"=w251) -> ("S"=w256:string)  [unwired: 10 in]
            n86 = Number To Fractional String(number=w250, precision (6)=i16 2) -> (F-format string=w260:string)  [unwired: 2 in]
            n87 = Build Array(w274, "Continuité" ("élément"), w263, w262) -> (w277:string[])
            n88 = Replace Array Subset(array=string[][] [["R continuité (Ohm)", "", "", "", "", "Vérification de la continuité par rapport à la masse"]] ("Tableau"), new element #1=w257, index (row) #1=w254, index (col) #1=1 ("disabled index (col)"), new element #2=w260, index (row) #2=w254, index (col) #2=3 ("disabled index (col)"), new element #3="0" ("nouvel élément/sous-tableau"), index (row) #3=w254, index (col) #3=2 ("disabled index (col)"), new element #4=w256, index (row) #4=w254, index (col) #4=4 ("disabled index (col)")) -> (w265:string[][])
            n89 = call "HTML_Table_Head.vi"("entrée d'erreur (pas d'erreur)"=w271, "Tableau"=w277, "chaîne en entrée"=w269) -> ("sortie d'erreur"=w276:errorcluster, "result string"=w275:string)  [unwired: 7 in]
            n90 = call "HTML_Table_Data.vi"("entrée d'erreur (pas d'erreur)"=w276, "Tableau"=w265, "chaîne en entrée"=w275) -> ("sortie d'erreur"=w270:errorcluster, "result string"=w266:string)  [unwired: 7 in]
          }
          frame "Iso+" {
            # "02/05/2023;Test# 1 ISO+/-"
            n91 = Index Array(array=w295) -> (element #3=w284:string, element #5=w283:string, element #7=w281:string, element #9=w282:string)  [unwired: 9 in, 5 out]
            n92 = Bundle(w284, w283, w281, w282) -> (w279:cluster{string, string, string, string})  [unwired: 1 in]
            n93 = call "OP600ZP_CLUSTER_ISO.vi"("Tableau 3"=string[][] [["R iso +(MOmhs)", "", "", "NA", "", "Résistance d'isolement BAT + / Chassis"], ["R iso - (MOhms)", "", "", "NA", "", "Résistance d'isolement BAT - / Chassis"]] ("Tableau"), "Numérique en entrée"=w292, "MESURES ISO"=w279) -> ("Chaîne"=w298:string, "Tableau 2"=w290:string[][], "Numérique en sortie"=w286:i32, "Tableau"=w289:bool[])  [unwired: 5 in]
            n94 = call <vilib>:"DataCell_NbPASSFAIL_Bool.vi"("Tableau en entrée"=w289) -> ("Chaîne"=w287:string, "Chaîne 2"=w288:string)  [unwired: 8 in, 1 out]
            n95 = Build Array(w298, "Isolement" ("élément"), w288, w287, "NA" ("élément")) -> (w301:string[])
            n96 = call "HTML_Table_Head.vi"("entrée d'erreur (pas d'erreur)"=w294, "Tableau"=w301, "chaîne en entrée"=w285) -> ("sortie d'erreur"=w300:errorcluster, "result string"=w299:string)  [unwired: 7 in]
            n97 = call "HTML_Table_Data.vi"("entrée d'erreur (pas d'erreur)"=w300, "Tableau"=w290, "chaîne en entrée"=w299) -> ("sortie d'erreur"=w293:errorcluster, "result string"=w291:string)  [unwired: 7 in]
          }
          frame "MCU" {
            n98 = Index Array(array=w330) -> (element #4=w314:string, element #6=w312:string, element #8=w313:string, element #10=w309:string, element #12=w308:string, element #14=w311:string, element #16=w310:string, element #18=w305:string, element #20=w303:string, element #22=w302:string)  [unwired: 22 in, 12 out]
            n99 = Bundle(w314, w309, w308, w311, w310, w313, w312, w305, w303, w302) -> (w304:T2)  [unwired: 1 in]
            n100 = call "OP600ZP_CLUSTER_SOFTS.vi"("MESURES"=w304, "EmptyTab"=string[][] [["Ubatt (V)", "", "", "", "", "Tension du Pack"], ["T Cell Max (°C)", "", "NA", "", "", "Température de cellule max mesurée"], ["T Cell Min (°C)", "", "", "NA", "", "Température de cellule min mesurée"], ["V Cell Max (mV)", "", "NA", "", "", "Tension de cellule max mesurée"], ["V Cell Min (mV)", "", "", "NA", "", "Tension de cellule min mesurée"], ["DeltaTCell (°C)", "", "NA", "", "", "Delta max de température mesuré"], ["DeltaVCell (mV)", "", "NA", "", "", "Delta max de tension mesuré"], ["TUsine (°C)", "", "", "", "", "Relevé de la température de l'usine"], ["SOC", "", "", "NA", "", "Seuil Of Charge"], ["SOH", "", "", "NA", "", "State Of Health"]] ("Tableau")) -> ("Tab1"=w307:string[][], "PASS/FAIL"=w306:bool[])  [unwired: 8 in]
            n101 = Increment(x=w322) -> (x+1=w321:i32)
            n102 = call <vilib>:"DataCell_NbPASSFAIL_Bool.vi"("Tableau en entrée"=w306) -> ("Chaîne"=w323:string, "Chaîne 2"=w324:string)  [unwired: 8 in, 1 out]
            n103 = Number To Decimal String(number=w321) -> (decimal integer string=w327:string)  [unwired: 1 in]
            n104 = Build Array(w327, "MCU" ("élément"), w324, w323, "NA" ("élément")) -> (w329:string[])
            n105 = call "HTML_Table_Head.vi"("entrée d'erreur (pas d'erreur)"=w318, "Tableau"=w329, "chaîne en entrée"=w315) -> ("sortie d'erreur"=w317:errorcluster, "result string"=w328:string)  [unwired: 7 in]
            n106 = call "HTML_Table_Data.vi"("entrée d'erreur (pas d'erreur)"=w317, "Tableau"=w307, "chaîne en entrée"=w328) -> ("sortie d'erreur"=w316:errorcluster, "result string"=w320:string)  [unwired: 7 in]
          }
          frame "OCV" {
            # "04/11/2022;Test# 3 - Vpack"
            n107 = Index Array(array=w344) -> (element #3=w334:string, element #5=w332:string)  [unwired: 6 in, 4 out]
            n108 = Bundle(w334, w332) -> (w333:cluster{string, string})  [unwired: 1 in]
            n109 = call "OP600ZP_CLUSTER_OCVACIR.vi"("MESURES_OCV"=w333, "Tableau 3"=string[][] [["Tension Pack (V)", "", "", "", "", "Tension du pack"], ["Ratio Ubatt/OCV", "", "NA", "", "", "Ratio Ubatt/OCV"]] ("Tableau")) -> ("Tableau"=w337:bool[], "Tableau 2"=w338:string[][])  [unwired: 8 in]
            n110 = Increment(x=w340) -> (x+1=w331:i32)
            n111 = call <vilib>:"DataCell_NbPASSFAIL_Bool.vi"("Tableau en entrée"=w337) -> ("Chaîne"=w335:string, "Chaîne 2"=w336:string)  [unwired: 8 in, 1 out]
            n112 = Number To Decimal String(number=w331) -> (decimal integer string=w347:string)  [unwired: 1 in]
            n113 = Build Array(w347, "OCV" ("élément"), w336, w335, "NA" ("élément")) -> (w350:string[])
            n114 = call "HTML_Table_Head.vi"("entrée d'erreur (pas d'erreur)"=w343, "Tableau"=w350, "chaîne en entrée"=w341) -> ("sortie d'erreur"=w349:errorcluster, "result string"=w348:string)  [unwired: 7 in]
            n115 = call "HTML_Table_Data.vi"("entrée d'erreur (pas d'erreur)"=w349, "Tableau"=w338, "chaîne en entrée"=w348) -> ("sortie d'erreur"=w342:errorcluster, "result string"=w339:string)  [unwired: 7 in]
          }
          frame "DTC" {
            w357 = 0 ("indice (ligne)")
            n116 = Index Array(array=w361) -> (element #3=w359:string)  [unwired: 3 in, 2 out]
            n117 = Equal?(x=w359, y="NO DTC") -> (x = y?=w354:bool)
            n118 = Build Array(w354) -> (w353:bool[])
            n119 = call <vilib>:"PASSFAIL.vi"("E"=w354) -> ("S"=w355:string)  [unwired: 10 in]
            n120 = Increment(x=w366) -> (x+1=w352:i32)
            n121 = call <vilib>:"DataCell_NbPASSFAIL_Bool.vi"("Tableau en entrée"=w353) -> ("Chaîne"=w369:string, "Chaîne 2"=w370:string)  [unwired: 8 in, 1 out]
            n122 = Number To Decimal String(number=w352) -> (decimal integer string=w373:string)  [unwired: 1 in]
            n123 = Build Array(w373, "DTC" ("élément"), w370, w369, "NA" ("élément")) -> (w376:string[])
            n124 = Replace Array Subset(array=string[][] [["DTC", "", "NA", "NA", "", "Vérification de la présence de DTC"]] ("Tableau"), new element #1=w359, index (row) #1=w357, index (col) #1=1 ("indice désactivé (col)"), new element #2=w355, index (row) #2=w357, index (col) #2=4 ("indice désactivé (col)")) -> (w364:string[][])
            n125 = call "HTML_Table_Head.vi"("entrée d'erreur (pas d'erreur)"=w368, "Tableau"=w376, "chaîne en entrée"=w362) -> ("sortie d'erreur"=w375:errorcluster, "result string"=w374:string)  [unwired: 7 in]
            n126 = call "HTML_Table_Data.vi"("entrée d'erreur (pas d'erreur)"=w375, "Tableau"=w364, "chaîne en entrée"=w374) -> ("sortie d'erreur"=w367:errorcluster, "result string"=w363:string)  [unwired: 7 in]
          }
          frame "DTC2" {
            w388 = 0 ("indice (ligne)")
            n127 = Index Array(array=w381) -> (element #3=w390:string)  [unwired: 3 in, 2 out]
            n128 = Equal?(x=w390, y="NO DTC") -> (x = y?=w385:bool)
            n129 = Build Array(w385) -> (w384:bool[])
            n130 = call <vilib>:"PASSFAIL.vi"("E"=w385) -> ("S"=w386:string)  [unwired: 10 in]
            n131 = Increment(x=w382) -> (x+1=w379:i32)
            n132 = call <vilib>:"DataCell_NbPASSFAIL_Bool.vi"("Tableau en entrée"=w384) -> ("Chaîne"=w394:string, "Chaîne 2"=w395:string)  [unwired: 8 in, 1 out]
            n133 = Number To Decimal String(number=w379) -> (decimal integer string=w398:string)  [unwired: 1 in]
            n134 = Build Array(w398, "DTC2" ("élément"), w395, w394, "NA" ("élément")) -> (w401:string[])
            n135 = Replace Array Subset(array=string[][] [["DTC2", "", "NA", "NA", "", "Vérification de la présence de DTC2"]] ("Tableau"), new element #1=w390, index (row) #1=w388, index (col) #1=1 ("indice désactivé (col)"), new element #2=w386, index (row) #2=w388, index (col) #2=4 ("indice désactivé (col)")) -> (w392:string[][])
            n136 = call "HTML_Table_Head.vi"("entrée d'erreur (pas d'erreur)"=w383, "Tableau"=w401, "chaîne en entrée"=w380) -> ("sortie d'erreur"=w400:errorcluster, "result string"=w399:string)  [unwired: 7 in]
            n137 = call "HTML_Table_Data.vi"("entrée d'erreur (pas d'erreur)"=w400, "Tableau"=w392, "chaîne en entrée"=w399) -> ("sortie d'erreur"=w378:errorcluster, "result string"=w377:string)  [unwired: 7 in]
          }
          frame "PARK" {
            n138 = Index Array(array=w417) -> (element #4=w402:string, element #6=w403:string, element #8=w410:string, element #10=w409:string, element #12=w408:string, element #14=w407:string, element #16=w404:string, element #18=w405:string)  [unwired: 23 in, 15 out]
            n139 = Bundle(w410, w409, w408, w407, w403, w402, w405, w404) -> (w406:T3)  [unwired: 1 in]
            n140 = call "OP600ZP_CLUSTER_SOFTS_FIN.vi"("MESURES"=w406, "EmptyTab"=string[][] [["T Cell Max (°C)", "", "NA", "", "", "Température de cellule max mesurée"], ["T Cell Min (°C)", "", "", "NA", "", "Température de cellule min mesurée"], ["V Cell Max (mV)", "", "NA", "", "", "Tension de cellule max mesurée"], ["V Cell Min (mV)", "", "", "NA", "", "Tension de cellule min mesurée"], ["DeltaTCell (°C)", "", "NA", "", "", "Delta max de température mesuré"], ["DeltaVCell (mV)", "", "NA", "", "", "Delta max de tension mesuré"], ["SOC", "", "", "", "", "Seuil Of Charge"], ["SOH", "", "", "NA", "", "State Of Health"]] ("Tableau")) -> ("Tab1"=w419:string[][], "PASS/FAIL"=w418:bool[])  [unwired: 8 in]
            n141 = Increment(x=w415) -> (x+1=w413:i32)
            n142 = call <vilib>:"DataCell_NbPASSFAIL_Bool.vi"("Tableau en entrée"=w418) -> ("Chaîne"=w422:string, "Chaîne 2"=w423:string)  [unwired: 8 in, 1 out]
            n143 = Number To Decimal String(number=w413) -> (decimal integer string=w426:string)  [unwired: 1 in]
            n144 = Build Array(w426, "PARK" ("élément"), w423, w422, "NA" ("élément")) -> (w428:string[])
            n145 = call "HTML_Table_Head.vi"("entrée d'erreur (pas d'erreur)"=w416, "Tableau"=w428, "chaîne en entrée"=w414) -> ("sortie d'erreur"=w420:errorcluster, "result string"=w427:string)  [unwired: 7 in]
            n146 = call "HTML_Table_Data.vi"("entrée d'erreur (pas d'erreur)"=w420, "Tableau"=w419, "chaîne en entrée"=w427) -> ("sortie d'erreur"=w412:errorcluster, "result string"=w411:string)  [unwired: 7 in]
          }
          frame "FIN_TEST" {
            w442 = "OK"
            n147 = Index Array(array=w468) -> (element #4=w445:string, element #6=w444:string, element #8=w443:string)  [unwired: 10 in, 7 out]
            n148 = Equal?(x=w445, y=w442) -> (x = y?=w440:bool)
            n149 = Equal?(x=w444, y=w442) -> (x = y?=w439:bool)
            n150 = Equal?(x=w443, y=w442) -> (x = y?=w438:bool)
            n151 = call <vilib>:"PASSFAIL.vi"("E"=w440) -> ("S"=w437:string)  [unwired: 10 in]
            n152 = call <vilib>:"PASSFAIL.vi"("E"=w439) -> ("S"=w436:string)  [unwired: 10 in]
            n153 = call <vilib>:"PASSFAIL.vi"("E"=w438) -> ("S"=w435:string)  [unwired: 10 in]
            n154 = Build Array(w440, w439, w438) -> (w441:bool[])
            n155 = Increment(x=w454) -> (x+1=w455:i32)
            n156 = call <vilib>:"DataCell_NbPASSFAIL_Bool.vi"("Tableau en entrée"=w441) -> ("Chaîne"=w460:string, "Chaîne 2"=w461:string)  [unwired: 8 in, 1 out]
            n157 = Number To Decimal String(number=w455) -> (decimal integer string=w464:string)  [unwired: 1 in]
            n158 = Replace Array Subset(array=string[][] [["Etiquettes", "", "NA", "NA", "", "Vérification de la présence des étiquettes"], ["Esthetique", "", "NA", "NA", "", "Vérification de l'ésthetique du pack"], ["VAT", "", "NA", "NA", "", "Vérification de l'absence de tension"]] ("Tableau"), new element #1=w445, index (row) #1=0 ("indice (ligne)"), index (col) #1=1 ("indice désactivé (col)"), new element #2=w444, index (row) #2=1 ("indice (ligne)"), index (col) #2=1 ("indice désactivé (col)"), new element #3=w443, index (row) #3=2 ("indice (ligne)"), index (col) #3=1 ("indice désactivé (col)"), new element #4=w437, index (row) #4=0 ("indice (ligne)"), index (col) #4=4 ("indice désactivé (col)"), new element #5=w436, index (row) #5=1 ("indice (ligne)"), index (col) #5=4 ("indice désactivé (col)"), new element #6=w435, index (row) #6=2 ("indice (ligne)"), index (col) #6=4 ("indice désactivé (col)")) -> (w452:string[][])
            n159 = Build Array(w464, "FIN_TEST" ("élément"), w461, w460, "NA" ("élément")) -> (w466:string[])
            n160 = call "HTML_Table_Head.vi"("entrée d'erreur (pas d'erreur)"=w458, "Tableau"=w466, "chaîne en entrée"=w453) -> ("sortie d'erreur"=w459:errorcluster, "result string"=w465:string)  [unwired: 7 in]
            n161 = call "HTML_Table_Data.vi"("entrée d'erreur (pas d'erreur)"=w459, "Tableau"=w452, "chaîne en entrée"=w465) -> ("sortie d'erreur"=w457:errorcluster, "result string"=w456:string)  [unwired: 7 in]
          }
          frame "Capacitance" {
            w489 = 1 ("indice désactivé (col)")
            n162 = global read "OP600ZP_VGConf.vi" "CBAT+"() -> (w497:dbl)
            n163 = global read "OP600ZP_VGConf.vi" "CBAT-"() -> (w496:dbl)
            n164 = global read "OP600ZP_VGConf.vi" "CBATmin"() -> (w474:dbl)
            n165 = Index Array(array=w516) -> (element #4=w486:string, element #6=w484:string)  [unwired: 6 in, 4 out]
            n166 = Number To Fractional String(number=w497, precision (6)=i16 2 ("précision (6)")) -> (F-format string=w485:string)  [unwired: 2 in]
            n167 = Number To Fractional String(number=w496, precision (6)=i16 2 ("précision (6)")) -> (F-format string=w483:string)  [unwired: 2 in]
            n168 = Number To Fractional String(number=w474, precision (6)=i16 2 ("précision (6)")) -> (F-format string=w469:string)  [unwired: 2 in]
            n169 = Less?(x=w484, y=w483) -> (x < y?=w478:bool)
            n170 = Less?(x=w486, y=w485) -> (x < y?=w477:bool)
            n171 = Build Array(w477, w478) -> (w476:bool[])
            n172 = call <vilib>:"PASSFAIL.vi"("E"=w478) -> ("S"=w487:string)  [unwired: 10 in]
            n173 = call <vilib>:"PASSFAIL.vi"("E"=w477) -> ("S"=w488:string)  [unwired: 10 in]
            n174 = Increment(x=w503) -> (x+1=w502:i32)
            n175 = call <vilib>:"DataCell_NbPASSFAIL_Bool.vi"("Tableau en entrée"=w476) -> ("Chaîne"=w505:string, "Chaîne 2"=w506:string)  [unwired: 8 in, 1 out]
            n176 = Number To Decimal String(number=w502) -> (decimal integer string=w509:string)  [unwired: 1 in]
            n177 = Replace Array Subset(array=string[][] [["CBAT+ (nF)", "", "", "", "", "Mesure capacité BAT+/châssis"], ["CBAT- (nF)", "", "", "", "", "Mesure capacité BAT-/châssis"]] ("Tableau"), new element #1=w486, index (row) #1=0 ("indice (ligne)"), index (col) #1=1 ("indice désactivé (col)"), new element #2=w484, index (row) #2=w489, index (col) #2=w489, new element #3=w485, index (row) #3=0 ("indice (ligne)"), index (col) #3=3 ("indice désactivé (col)"), new element #4=w483, index (row) #4=1 ("indice (ligne)"), index (col) #4=3 ("indice désactivé (col)"), new element #5=w488, index (row) #5=0 ("indice (ligne)"), index (col) #5=4 ("indice désactivé (col)"), new element #6=w487, index (row) #6=1 ("indice (ligne)"), index (col) #6=4 ("indice désactivé (col)"), new element #7=w469, index (row) #7=0 ("indice (ligne)"), index (col) #7=2 ("indice désactivé (col)"), new element #8=w469, index (row) #8=1 ("indice (ligne)"), index (col) #8=2 ("indice désactivé (col)")) -> (w500:string[][])
            n178 = Build Array(w509, "Capacité" ("élément"), w506, w505, "NA" ("élément")) -> (w512:string[])
            n179 = call "HTML_Table_Head.vi"("entrée d'erreur (pas d'erreur)"=w504, "Tableau"=w512, "chaîne en entrée"=w501) -> ("sortie d'erreur"=w511:errorcluster, "result string"=w510:string)  [unwired: 7 in]
            n180 = call "HTML_Table_Data.vi"("entrée d'erreur (pas d'erreur)"=w511, "Tableau"=w500, "chaîne en entrée"=w510) -> ("sortie d'erreur"=w499:errorcluster, "result string"=w498:string)  [unwired: 7 in]
          }
          frame "INTERLOOP" {
            w524 = "NO DTC" ("x")
            w550 = "DTC" ("x")
            n181 = Index Array(array=w571) -> (element #4=w551:string, element #6=w549:string, element #8=w548:string, element #10=w547:string, element #12=w521:string)  [unwired: 12 in, 7 out]
            n182 = Equal?(x=w550, y=w551) -> (x = y?=w546:bool)
            n183 = Equal?(x=w549, y=w550) -> (x = y?=w545:bool)
            n184 = Equal?(x=w550, y=w548) -> (x = y?=w544:bool)
            n185 = Equal?(x=w524, y=w547) -> (x = y?=w543:bool)
            n186 = Equal?(x=w524, y=w521) -> (x = y?=w522:bool)
            n187 = Build Array(w546, w545, w544, w543, w522) -> (w560:bool[])
            n188 = call <vilib>:"PASSFAIL.vi"("E"=w522) -> ("S"=w523:string)  [unwired: 10 in]
            n189 = call <vilib>:"PASSFAIL.vi"("E"=w546) -> ("S"=w542:string)  [unwired: 10 in]
            n190 = call <vilib>:"PASSFAIL.vi"("E"=w545) -> ("S"=w541:string)  [unwired: 10 in]
            n191 = call <vilib>:"PASSFAIL.vi"("E"=w544) -> ("S"=w540:string)  [unwired: 10 in]
            n192 = call <vilib>:"PASSFAIL.vi"("E"=w543) -> ("S"=w539:string)  [unwired: 10 in]
            n193 = Increment(x=w528) -> (x+1=w525:i32)
            n194 = call <vilib>:"DataCell_NbPASSFAIL_Bool.vi"("Tableau en entrée"=w560) -> ("Chaîne"=w562:string, "Chaîne 2"=w563:string)  [unwired: 8 in, 1 out]
            n195 = Number To Decimal String(number=w525) -> (decimal integer string=w566:string)  [unwired: 1 in]
            n196 = Replace Array Subset(array=string[][] [["X & Y débranchés", "", "NA", "NA", "", "Connecteurs de puissance X & Y débranchés"], ["Y débranché", "", "NA", "NA", "", "Connecteur de puissance Y débranché"], ["X débranché", "", "NA", "NA", "", "Connecteur de puissance X débranché"], ["X & Y branchés", "", "NA", "NA", "", "Connecteurs de puissance X & Y branchés"], ["DTC DRIVE", "", "NA", "NA", "", "Vérifie la présence de DTC en mode DRIVE"]] ("Tableau"), new element #1=w551, index (row) #1=0 ("indice (ligne)"), index (col) #1=1 ("indice désactivé (col)"), new element #2=w549, index (row) #2=1 ("indice (ligne)"), index (col) #2=1 ("indice désactivé (col)"), new element #3=w548, index (row) #3=2 ("indice (ligne)"), index (col) #3=1 ("indice désactivé (col)"), new element #4=w547, index (row) #4=3 ("indice (ligne)"), index (col) #4=1 ("indice désactivé (col)"), new element #5=w542, index (row) #5=0 ("indice (ligne)"), index (col) #5=4 ("indice désactivé (col)"), new element #6=w541, index (row) #6=1 ("indice (ligne)"), index (col) #6=4 ("indice désactivé (col)"), new element #7=w540, index (row) #7=2 ("indice (ligne)"), index (col) #7=4 ("indice désactivé (col)"), new element #8=w539, index (row) #8=3 ("indice (ligne)"), index (col) #8=4 ("indice désactivé (col)"), new element #9=w521, index (row) #9=4 ("indice (ligne)"), index (col) #9=1 ("indice désactivé (col)"), new element #10=w523, index (row) #10=4 ("indice (ligne)"), index (col) #10=4 ("indice désactivé (col)")) -> (w561:string[][])
            n197 = Build Array(w566, "INTERLOOP" ("élément"), w563, w562, "NA" ("élément")) -> (w569:string[])
            n198 = call "HTML_Table_Head.vi"("entrée d'erreur (pas d'erreur)"=w527, "Tableau"=w569, "chaîne en entrée"=w526) -> ("sortie d'erreur"=w568:errorcluster, "result string"=w567:string)  [unwired: 7 in]
            n199 = call "HTML_Table_Data.vi"("entrée d'erreur (pas d'erreur)"=w568, "Tableau"=w561, "chaîne en entrée"=w567) -> ("sortie d'erreur"=w529:errorcluster, "result string"=w530:string)  [unwired: 7 in]
          }
          frame "PreCharge" {
            n200 = Index Array(array=w589) -> (element #6=w572:string)  [unwired: 8 in, 7 out]
            n201 = Increment(x=w579) -> (x+1=w574:i32)
            n202 = Number To Decimal String(number=w574) -> (decimal integer string=w584:string)  [unwired: 1 in]
            n203 = call "OP600ZP_PreCharge.vi"("PR"=w572, "Tableau en entrée"=string[][] [["UFinal (V)", "", "", "", "", "Tension capacité"]] ("Tableau")) -> ("Tableau en sortie"=w577:string[][], "PASS?"=w573:bool[])  [unwired: 8 in]
            n204 = call <vilib>:"DataCell_NbPASSFAIL_Bool.vi"("Tableau en entrée"=w573) -> ("Chaîne"=w581:string, "Chaîne 2"=w582:string)  [unwired: 8 in, 1 out]
            n205 = Build Array(w584, "PreCharge" ("élément"), w582, w581) -> (w587:string[])
            n206 = call "HTML_Table_Head.vi"("entrée d'erreur (pas d'erreur)"=w580, "Tableau"=w587, "chaîne en entrée"=w578) -> ("sortie d'erreur"=w586:errorcluster, "result string"=w585:string)  [unwired: 7 in]
            n207 = call "HTML_Table_Data.vi"("entrée d'erreur (pas d'erreur)"=w586, "Tableau"=w577, "chaîne en entrée"=w585) -> ("sortie d'erreur"=w575:errorcluster, "result string"=w576:string)  [unwired: 7 in]
          }
          frame "Current + DCIR" {
            n208 = Index Array(array=w615) -> (element #4=w600:string, element #6=w599:string, element #8=w598:string, element #12=w597:string, element #14=w596:string, element #16=w595:string, element #18=w591:string, element #20=w590:string)  [unwired: 20 in, 12 out]
            n209 = Bundle(w600, w599, w598, w597, w596, w595, w591, w590) -> (w594:T3)  [unwired: 1 in]
            n210 = Increment(x=w605) -> (x+1=w604:i32)
            n211 = Number To Decimal String(number=w604) -> (decimal integer string=w611:string)  [unwired: 1 in]
            n212 = call "OP600ZP_DCIR.vi"("tableau"=string[][] [["Current@0s (mA)", "", "NA", "", "", "Courant à t=0s"], ["DeltaV@0s (mV)", "", "NA", "", "", "Delta max de tension mesuré (T=0s)"], ["DeltaT@0s (°C)", "", "NA", "", "", "Delta max de température mesuré (T=0s)"], ["Current@30s (A)", "", "", "", "", "Courant à t=30s"], ["DeltaV@30s (mV)", "", "NA", "", "", "Delta max de tension mesuré (T=30s)"], ["DeltaT@30s (°C)", "", "NA", "", "", "Delta max de température mesuré (T=30s)"], ["DCIR@1C (mOhms)", "", "NA", "", "", "Mesure de la résistance interne"], ["Delta²V", "", "NA", "", "", "Delta de tension entre DeltaV@0s et DeltaV@30s"], ["Delta²T", "", "NA", "", "", "Delta de tension entre DeltaT@0s et DeltaT@30s"], ["UPostRelax (V)", "", "", "", "", "Tension post relaxation"]] ("Tableau"), "DCIR_MESURES"=w594) -> ("Tableau 2"=w603:string[][], "PASS/FAIL"=w601:bool[])  [unwired: 8 in]
            n213 = call <vilib>:"DataCell_NbPASSFAIL_Bool.vi"("Tableau en entrée"=w601) -> ("Chaîne"=w608:string, "Chaîne 2"=w609:string)  [unwired: 8 in, 1 out]
            n214 = Build Array(w611, "DCIR" ("élément"), w609, w608) -> (w614:string[])
            n215 = call "HTML_Table_Head.vi"("entrée d'erreur (pas d'erreur)"=w607, "Tableau"=w614, "chaîne en entrée"=w593) -> ("sortie d'erreur"=w613:errorcluster, "result string"=w612:string)  [unwired: 7 in]
            n216 = call "HTML_Table_Data.vi"("entrée d'erreur (pas d'erreur)"=w613, "Tableau"=w603, "chaîne en entrée"=w612) -> ("sortie d'erreur"=w606:errorcluster, "result string"=w602:string)  [unwired: 7 in]
          }
          frame "NULL", Default {
            # "NULL"
          }
        }
      }
    }
  }
  n217 = Concatenate Strings(w12, "\\" ("chaîne"), w10) -> (w9:string)
  n218 = String To Path(string=w9) -> (path=w15:path)
  "network out" <- w15
  n219 = Search and Replace String(replace all?=TRUE ("tout remplacer ? (F)"), input string=w49, search string="<td class=\"core1 testpass\">FAIL</td>" ("chaîne recherchée"), replace string="<td class=\"core1 testfail\">FAIL</td>" ("chaîne de remplacement (\"\")"), error in=w47) -> (result string=w33:string, number of replacements=w28:i32, error out=w44:errorcluster)  [unwired: 3 in, 1 out]
  n220 = Search and Replace String(replace all?=TRUE ("tout remplacer ? (F)"), input string=w33, search string="<td class=\"core1 testpass\">PASS</td>" ("chaîne recherchée"), error in=w44) -> (number of replacements=w36:i32, error out=w40:errorcluster)  [unwired: 4 in, 2 out]
  "nombre de remplacements" <- w36
  n221 = Number To Decimal String(number=w36) -> (decimal integer string=w35:string)  [unwired: 1 in]
  n222 = Number To Decimal String(number=w28) -> (decimal integer string=w34:string)  [unwired: 1 in]
  n223 = Search and Replace String(input string=w33, search string="<!--NBTESTOK-->" ("chaîne recherchée"), replace string=w35, error in=w40) -> (result string=w41:string, error out=w39:errorcluster)  [unwired: 4 in, 2 out]
  n224 = Equal To 0?(x=w28) -> (x = 0?=w20:bool)
  n225 = Search and Replace String(input string=w41, search string="<!--NBTESTKO-->" ("chaîne recherchée"), replace string=w34, error in=w39) -> (result string=w23:string, error out=w27:errorcluster)  [unwired: 4 in, 2 out]
  n226 = Search and Replace String(input string=w23, search string="Résultat du test :\t</td><td class=\"resume5\" colspan=\"3\"><div><span style=\"float:left\" id=\"result\"><font size = \"5pt\" color=\"green\"><b>CONFORME</b>", replace string="Résultat du test :\t</td><td class=\"resume5\" colspan=\"3\"><div><span style=\"float:left\" id=\"result\"><font  size = \"5pt\" color=\"red\"><b>NON CONFORME</b>", error in=w27) -> (result string=w5:string, error out=w26:errorcluster)  [unwired: 4 in, 2 out]
  n227 = Search and Replace String(input string=w5, search string=".resume1,.resume3,.resume4,.resume5,.resume6,.resume7{background-color:#e6feef;padding:7px;border:1px solid black;}\n.resume0{border:1px solid black;background-color:#e6feef;font-weight: bold;padding:0px;text-align: center;}", replace string=".resume1,.resume3,.resume4,.resume5,.resume6,.resume7{background-color:#fdebd0;padding:7px;border:1px solid black;}\n.resume0{border:1px solid black;background-color:#fdebd0;font-weight: bold;padding:0px;text-align: center;}") -> (result string=w4:string)  [unwired: 5 in, 3 out]
  n228 = Select(t=w23, s=w20, f=w4) -> (s? t:f=w24:string)
  "Chaîne" <- w24
  n229 = Not Equal?(x=w15, y=path "") -> (x != y?=w17:bool)
  n230 = Open/Create/Replace File(file path (use dialog)=w50, error in=w26, operation (0:open)=w32) -> (refnum out=w56:refnum<file>, error out=w58:errorcluster)  [unwired: 3 in, 1 out]
  n231 = case shown="Vrai" w17 {
    tunnel: w32 -> [_ w624]
    tunnel: w15 -> [_ w623]
    tunnel: w26 -> [_ w622]
    tunnel: w24 -> [_ w621]
    tunnel: [errorcluster {"status"=FALSE, "code"=0, "source"=""} ("error out") w620] -> w22
    frame False {
    }
    frame True {
      n232 = Open/Create/Replace File(file path (use dialog)=w623, error in=w622, operation (0:open)=w624) -> (refnum out=w625:refnum<file>, error out=w627:errorcluster)  [unwired: 3 in, 1 out]
      n233 = Write to Text File(file (use dialog)=w625, text=w621, error in=w627) -> (refnum out=w626:refnum<file>, error out=w628:errorcluster)  [unwired: 1 in, 1 out]
      n234 = Close File(refnum=w626, error in=w628) -> (error out=w620:errorcluster)  [unwired: 1 out]
    }
  }
  n235 = Write to Text File(file (use dialog)=w56, text=w24, error in=w58) -> (refnum out=w57:refnum<file>, error out=w59:errorcluster)  [unwired: 1 in, 1 out]
  n236 = Close File(refnum=w57, error in=w59) -> (error out=w21:errorcluster)  [unwired: 1 out]
  n237 = Merge Errors(w21, w22) -> (w19:errorcluster)
  "sortie d'erreur" <- w19
  n238 = Compound Arithmetic op=AND ("Opérateur arithmétique")(w20, invert w19) -> (→"tout bon":bool)
